vi "CMD_Loop.vi"() -> ()   [LabVIEW 2020, in "2023-Auto_CMD.lvlib"]
uses:
  2023-Auto_CMD.lvlib
  Cluster_CMD_CMD_Data.ctl
  Shared Code/TypeDefs/ENUM_AutoSelect.ctl
  Shared Code/TypeDefs/Cluster_Auto Sequence Data.ctl
  ENUM_CMD_State.ctl
  Shared Code/TypeDefs/Cluster_Auto Sequence Settings.ctl
  ENUM_Drive Mode Select.ctl
  Shared Code/TypeDefs/Dial_Compase heading unit circle CCW positive.ctl
  MotionMaser/ENUM_Pose List.ctl
  Shared Code/TypeDefs/ENUM_Grabber_CMD_Mode Select.ctl
  Shared Code/TypeDefs/Cluster_Extend_SW Output Data.ctl
  Shared Code/TypeDefs/Cluster_Sholder_SW Output Data.ctl
  Sholder/Cluster_CMD_ACT_Data.ctl
  Shared Code/TypeDefs/ENUM_Sholder_CMD_Mode Select.ctl
  SwerveDrive/Cluster_CMD_ACT_Data.ctl
  Shared Code/TypeDefs/ENUM_Swerve_CMD_Mode Select.ctl
  Shared Code/TypeDefs/Cluster_CMD_Direction Data.ctl
  Shared Code/TypeDefs/Cluster_Module Velocity-Direction-Rotations.ctl
  Shared Code/TypeDefs/Level_Velocity plus-minus 1.ctl
  Type Defs/NUM_Rotate Input.ctl
  Shared Code/TypeDefs/Cluster_X-Y.ctl
  Grabber/Cluster_CMD_ACT_Data.ctl
  Extention/Cluster_CMD_ACT_Data.ctl
  Shared Code/TypeDefs/ENUM_Extend_CMD_Mode Select.ctl
  Wrist/Cluster_CMD_ACT_Data.ctl
  Shared Code/TypeDefs/ENUM_Wrist_CMD_Mode Select.ctl
  PigeonIMU/Cluster_CMD_SEN_Data.ctl
  Shared Code/TypeDefs/Cluster_Wrist_SW Output Data.ctl
  ENUM_CMD_Action.ctl
  Shared Code/TypeDefs/Cluster_AutoSequence.ctl
  Type Defs/Cluster_Pigeon Tilt Data.ctl
  Shared Code/TypeDefs/ENUM_Tilt State.ctl
  Shared Code/TypeDefs/Cluster_Grabber_SW Outputs.ctl
  <vilib>/Rock Robotics/WPI/DriverStation/WPI_DriverStationRobotMode2.ctl
  Shared Code/TypeDefs/Cluster_Config_AutoData.ctl
  fdd46993-b9fc-440f-aafb-7ab1a8c35176.vi
  133b30be-2fcb-456e-b4b0-07f770c500ae.vi
  1ba0cf27-86ce-4142-8b65-bcb405614ff3.vi
  09229b25-3731-4416-b61c-801146eec302.vi
  c7d6c6c0-b27b-4b8b-8552-511dbe9cf3c3.vi
  dfaa9063-9cc7-40d1-a81d-c10c38088b54.vi
  fdd46993-b9fc-440f-aafb-7ab1a8c35176.vi/f38ca901-adc1-4ad8-996e-31aeb746ae36.vi
  fdd46993-b9fc-440f-aafb-7ab1a8c35176.vi/958b2683-dd4b-41b7-8ed1-41c95f63cef0.vi
  133b30be-2fcb-456e-b4b0-07f770c500ae.vi/f38ca901-adc1-4ad8-996e-31aeb746ae36.vi
  133b30be-2fcb-456e-b4b0-07f770c500ae.vi/958b2683-dd4b-41b7-8ed1-41c95f63cef0.vi
  09229b25-3731-4416-b61c-801146eec302.vi/f38ca901-adc1-4ad8-996e-31aeb746ae36.vi
  09229b25-3731-4416-b61c-801146eec302.vi/958b2683-dd4b-41b7-8ed1-41c95f63cef0.vi
  c7d6c6c0-b27b-4b8b-8552-511dbe9cf3c3.vi/f38ca901-adc1-4ad8-996e-31aeb746ae36.vi
  c7d6c6c0-b27b-4b8b-8552-511dbe9cf3c3.vi/958b2683-dd4b-41b7-8ed1-41c95f63cef0.vi
  fdd46993-b9fc-440f-aafb-7ab1a8c35176.vi/f38ca901-adc1-4ad8-996e-31aeb746ae36.vi/1c6bd52c-bbca-4d4a-a290-93ea2703fded.vi
  fdd46993-b9fc-440f-aafb-7ab1a8c35176.vi/f38ca901-adc1-4ad8-996e-31aeb746ae36.vi/47c2b0d5-b5fa-444e-9535-611565d375db.vi
  133b30be-2fcb-456e-b4b0-07f770c500ae.vi/f38ca901-adc1-4ad8-996e-31aeb746ae36.vi/1c6bd52c-bbca-4d4a-a290-93ea2703fded.vi
  133b30be-2fcb-456e-b4b0-07f770c500ae.vi/f38ca901-adc1-4ad8-996e-31aeb746ae36.vi/47c2b0d5-b5fa-444e-9535-611565d375db.vi
  09229b25-3731-4416-b61c-801146eec302.vi/f38ca901-adc1-4ad8-996e-31aeb746ae36.vi/1c6bd52c-bbca-4d4a-a290-93ea2703fded.vi
  09229b25-3731-4416-b61c-801146eec302.vi/f38ca901-adc1-4ad8-996e-31aeb746ae36.vi/47c2b0d5-b5fa-444e-9535-611565d375db.vi
  c7d6c6c0-b27b-4b8b-8552-511dbe9cf3c3.vi/f38ca901-adc1-4ad8-996e-31aeb746ae36.vi/1c6bd52c-bbca-4d4a-a290-93ea2703fded.vi
  c7d6c6c0-b27b-4b8b-8552-511dbe9cf3c3.vi/f38ca901-adc1-4ad8-996e-31aeb746ae36.vi/47c2b0d5-b5fa-444e-9535-611565d375db.vi
  Robot Global Data.vi
  Utility/Global_STOP.vi
  <vilib>/Utility/Data Type/Get Type Information.vi
  <vilib>/Utility/error.llb/Trim Whitespace.vi
  Shared Code/Utility/RWA/RWA/File/RWA_PC FIle Read String.vi
  Shared Code/Utility/RWA/RWA/Read Write Anything/RWA_File String.vi
  Shared Code/Utility/RWA/RWA/File/RWA_PC File Write String.vi
  Wrist/Global_CMD_ACT_Data In.vi
  Extention/Global_CMD_ACT_Data In.vi
  Grabber/Global_CMD_ACT_Data In.vi
  PigeonIMU/Global_CMD_SEN_Data In.vi
  SwerveDrive/Global_CMD_ACT_Data In.vi
  Sholder/Global_CMD_ACT_Data In.vi
  Global_CMD_CMD_Data In.vi
  Sholder/Global_ACT_Data Out.vi
  Extention/Global_ACT_Data Out.vi
  SwerveDrive/Global_ACT_Data Out.vi
  Grabber/Global_ACT_Data Out.vi
  Wrist/Global_ACT_Data Out.vi
  PigeonIMU/Global_SEN_Data Out.vi
  Global_CMD_Data Out.vi
  <vilib>/Comparison/Equal/Equal Functor/Equal Functor.lvclass
  PigeonIMU/PigeonIMU_SEN.lvlib
  Sholder/Sholder_ACT.lvlib
  SwerveDrive/SwerveDrive_ACT.lvlib
  Extention/Extend_ACT.lvlib
  Grabber/Grabber_ACT.lvlib
  Wrist/Wrist_ACT.lvlib
  MotionMaser/MotionMaster_SubCMD.lvlib
panel:
  out "Swerve_Position ft":dbl
  out "Remaing Match Time":sgl
  out "Sen_Pigeon_Tilt Data":T1
  out "Step Index 2":i32
  out "CMD Input.Auto Select":T3=enum."Drop Mid Drive Straight"
  out "Found":bool
  out "Error Out":errorcluster
  out "Message Out":string
  in  "Read Saved Config":bool
  in  "Update Config":bool
  in  "Sequences":T4[](array[typedef])=[{"Name"=enum."Score Mid Over and Balance", "List"=[{"State"=enum."Moving Arm", "Max Wait Time (S)"=1.5, "CMDs"={"Drive Mode"=enum."Coast", "Auto Angle"=0.0, "Auto Target (ft)"=0.0, "Max speed ft/s"=0.0, "Arm Pose "=enum."Safe Position", "Grabber CMD"=enum."STOP"}, "Color Box"=0}, {"State"=enum."Moving Arm", "Max Wait Time (S)"=3.0, "CMDs"={"Drive Mode"=enum."Coast", "Auto Angle"=0.0, "Auto Target (ft)"=0.0, "Max speed ft/s"=0.0, "Arm Pose "=enum."Score Mid", "Grabber CMD"=enum."STOP"}, "Color Box"=10309376}, {"State"=enum."Grabbing", "Max Wait Time (S)"=0.2, "CMDs"={"Drive Mode"=enum."To Position", "Auto Angle"=0.0, "Auto Target (ft)"=10.0, "Max speed ft/s"=12.0, "Arm Pose "=enum."Score Mid", "Grabber CMD"=enum."Eject"}, "Color Box"=16711680}, {"State"=enum."Tilt UP or Position", "Max Wait Time (S)"=8.0, "CMDs"={"Drive Mode"=enum."To Position", "Auto Angle"=0.5, "Auto Target (ft)"=6.0, "Max speed ft/s"=14.0, "Arm Pose "=enum."Home Pos", "Grabber CMD"=enum."STOP"}, "Color Box"=16744448}, {"State"=enum."Driving to Position", "Max Wait Time (S)"=10.0, "CMDs"={"Drive Mode"=enum."To Position", "Auto Angle"=0.5, "Auto Target (ft)"=14.0, "Max speed ft/s"=10.0, "Arm Pose "=enum."Home Pos", "Grabber CMD"=enum."STOP"}, "Color Box"=16776960}, {"State"=enum."Driving to Position", "Max Wait Time (S)"=3.0, "CMDs"={"Drive Mode"=enum."To Position", "Auto Angle"=0.0, "Auto Target (ft)"=6.0, "Max speed ft/s"=13.0, "Arm Pose "=enum."Home Pos", "Grabber CMD"=enum."STOP"}, "Color Box"=6618880}, {"State"=enum."Balancing Level", "Max Wait Time (S)"=100.0, "CMDs"={"Drive Mode"=enum."Balance on Charger", "Auto Angle"=0.0, "Auto Target (ft)"=0.0, "Max speed ft/s"=10.0, "Arm Pose "=enum."None-Unknown", "Grabber CMD"=enum."STOP"}, "Color Box"=16860}]}, {"Name"=enum."Drop Mid Drive Straight", "List"=[{"State"=enum."Moving Arm", "Max Wait Time (S)"=1.5, "CMDs"={"Drive Mode"=enum."Coast", "Auto Angle"=0.0, "Auto Target (ft)"=0.0, "Max speed ft/s"=0.0, "Arm Pose "=enum."Safe Position", "Grabber CMD"=enum."STOP"}, "Color Box"=0}, {"State"=enum."Moving Arm", "Max Wait Time (S)"=4.0, "CMDs"={"Drive Mode"=enum."Coast", "Auto Angle"=0.0, "Auto Target (ft)"=0.0, "Max speed ft/s"=0.0, "Arm Pose "=enum."Score Mid", "Grabber CMD"=enum."STOP"}, "Color Box"=10309376}, {"State"=enum."Grabbing", "Max Wait Time (S)"=0.5, "CMDs"={"Drive Mode"=enum."To Position", "Auto Angle"=0.0, "Auto Target (ft)"=0.0, "Max speed ft/s"=0.0, "Arm Pose "=enum."Score Mid", "Grabber CMD"=enum."Eject"}, "Color Box"=16711680}, {"State"=enum."Driving to Position", "Max Wait Time (S)"=10.0, "CMDs"={"Drive Mode"=enum."To Position", "Auto Angle"=0.5, "Auto Target (ft)"=15.0, "Max speed ft/s"=16.0, "Arm Pose "=enum."Safe Position", "Grabber CMD"=enum."STOP"}, "Color Box"=16744448}, {"State"=enum."Moving Arm", "Max Wait Time (S)"=10.0, "CMDs"={"Drive Mode"=enum."Rotation Absolute", "Auto Angle"=0.0, "Auto Target (ft)"=0.0, "Max speed ft/s"=0.0, "Arm Pose "=enum."Safe Position", "Grabber CMD"=enum."STOP"}, "Color Box"=16776960}]}, {"Name"=enum."Drop mid dock and engage", "List"=[{"State"=enum."Moving Arm", "Max Wait Time (S)"=1.5, "CMDs"={"Drive Mode"=enum."Coast", "Auto Angle"=0.0, "Auto Target (ft)"=0.0, "Max speed ft/s"=0.0, "Arm Pose "=enum."Safe Position", "Grabber CMD"=enum."STOP"}, "Color Box"=0}, {"State"=enum."Moving Arm", "Max Wait Time (S)"=4.0, "CMDs"={"Drive Mode"=enum."Coast", "Auto Angle"=0.0, "Auto Target (ft)"=0.0, "Max speed ft/s"=0.0, "Arm Pose "=enum."Score Mid", "Grabber CMD"=enum."STOP"}, "Color Box"=10309376}, {"State"=enum."Grabbing", "Max Wait Time (S)"=0.2, "CMDs"={"Drive Mode"=enum."Coast", "Auto Angle"=0.0, "Auto Target (ft)"=0.0, "Max speed ft/s"=0.0, "Arm Pose "=enum."Score Mid", "Grabber CMD"=enum."Eject"}, "Color Box"=16711680}, {"State"=enum."Driving to Position", "Max Wait Time (S)"=4.0, "CMDs"={"Drive Mode"=enum."To Position", "Auto Angle"=0.5, "Auto Target (ft)"=6.0, "Max speed ft/s"=10.0, "Arm Pose "=enum."Home Pos", "Grabber CMD"=enum."STOP"}, "Color Box"=16744448}, {"State"=enum."Balancing Level", "Max Wait Time (S)"=100.0, "CMDs"={"Drive Mode"=enum."Balance on Charger", "Auto Angle"=0.4996, "Auto Target (ft)"=0.0, "Max speed ft/s"=10.0, "Arm Pose "=enum."Home Pos", "Grabber CMD"=enum."STOP"}, "Color Box"=16776960}]}, {"Name"=enum."Drop High dock and engage", "List"=[{"State"=enum."Grabbing", "Max Wait Time (S)"=0.2, "CMDs"={"Drive Mode"=enum."Coast", "Auto Angle"=0.0, "Auto Target (ft)"=0.0, "Max speed ft/s"=0.0, "Arm Pose "=enum."Score Mid", "Grabber CMD"=enum."STOP"}, "Color Box"=0}, {"State"=enum."Driving to Position", "Max Wait Time (S)"=5.0, "CMDs"={"Drive Mode"=enum."To Position", "Auto Angle"=0.5, "Auto Target (ft)"=15.0, "Max speed ft/s"=10.0, "Arm Pose "=enum."Score High", "Grabber CMD"=enum."STOP"}, "Color Box"=10309376}, {"State"=enum."Driving to Position", "Max Wait Time (S)"=3.0, "CMDs"={"Drive Mode"=enum."Coast", "Auto Angle"=0.0, "Auto Target (ft)"=10.0, "Max speed ft/s"=16.0, "Arm Pose "=enum."Score High", "Grabber CMD"=enum."Eject"}, "Color Box"=16711680}, {"State"=enum."Balancing Level", "Max Wait Time (S)"=100.0, "CMDs"={"Drive Mode"=enum."To Position", "Auto Angle"=0.5, "Auto Target (ft)"=6.0, "Max speed ft/s"=16.0, "Arm Pose "=enum."Home Pos", "Grabber CMD"=enum."STOP"}, "Color Box"=16744448}, {"State"=enum."Idling", "Max Wait Time (S)"=5.0, "CMDs"={"Drive Mode"=enum."Coast", "Auto Angle"=0.0, "Auto Target (ft)"=0.0, "Max speed ft/s"=0.0, "Arm Pose "=enum."None-Unknown", "Grabber CMD"=enum."STOP"}, "Color Box"=16776960}]}, {"Name"=enum."Drop Low dock and engage", "List"=[{"State"=enum."Grabbing", "Max Wait Time (S)"=0.5, "CMDs"={"Drive Mode"=enum."Coast", "Auto Angle"=0.0, "Auto Target (ft)"=0.0, "Max speed ft/s"=0.0, "Arm Pose "=enum."Home Pos", "Grabber CMD"=enum."Eject"}, "Color Box"=0}, {"State"=enum."Driving to Position", "Max Wait Time (S)"=4.0, "CMDs"={"Drive Mode"=enum."To Position", "Auto Angle"=0.5, "Auto Target (ft)"=9.0, "Max speed ft/s"=10.0, "Arm Pose "=enum."Home Pos", "Grabber CMD"=enum."STOP"}, "Color Box"=10309376}, {"State"=enum."Balancing Level", "Max Wait Time (S)"=100.0, "CMDs"={"Drive Mode"=enum."Balance on Charger", "Auto Angle"=0.5, "Auto Target (ft)"=0.0, "Max speed ft/s"=5.0, "Arm Pose "=enum."Home Pos", "Grabber CMD"=enum."STOP"}, "Color Box"=16711680}]}, {"Name"=enum."Over and Rebalance", "List"=[{"State"=enum."Grabbing", "Max Wait Time (S)"=0.2, "CMDs"={"Drive Mode"=enum."Coast", "Auto Angle"=0.0, "Auto Target (ft)"=0.0, "Max speed ft/s"=0.0, "Arm Pose "=enum."Home Pos", "Grabber CMD"=enum."Eject"}, "Color Box"=0}, {"State"=enum."Tilt UP or Position", "Max Wait Time (S)"=8.0, "CMDs"={"Drive Mode"=enum."To Position", "Auto Angle"=0.5, "Auto Target (ft)"=6.0, "Max speed ft/s"=12.0, "Arm Pose "=enum."Home Pos", "Grabber CMD"=enum."STOP"}, "Color Box"=10309376}, {"State"=enum."Driving to Position", "Max Wait Time (S)"=10.0, "CMDs"={"Drive Mode"=enum."To Position", "Auto Angle"=0.5, "Auto Target (ft)"=14.0, "Max speed ft/s"=9.0, "Arm Pose "=enum."Home Pos", "Grabber CMD"=enum."STOP"}, "Color Box"=16711680}, {"State"=enum."Driving to Position", "Max Wait Time (S)"=3.0, "CMDs"={"Drive Mode"=enum."To Position", "Auto Angle"=0.0, "Auto Target (ft)"=6.0, "Max speed ft/s"=13.0, "Arm Pose "=enum."Home Pos", "Grabber CMD"=enum."STOP"}, "Color Box"=16744448}, {"State"=enum."Balancing Level", "Max Wait Time (S)"=100.0, "CMDs"={"Drive Mode"=enum."Balance on Charger", "Auto Angle"=0.0, "Auto Target (ft)"=0.0, "Max speed ft/s"=10.0, "Arm Pose "=enum."Home Pos", "Grabber CMD"=enum."STOP"}, "Color Box"=16776960}]}] {"List"."CMDs"."Auto Angle" scale format="%.3f"}
  out "Balanced":bool
  out "Action":T12
  out "State":T6
  out "ACT_Wrist_SW Out":T13
  out "CMD_SEN_Pigeon_CMD":T14
  out "CMD_ACT_Wrist":T15
  out "Drive At Angle":bool
  out "Step Index":i32
  out "CMD_CMD_2022-Auto_Data":T17={"Auto Select"=enum."Drop mid dock and engage"}
  out "CMD_ACT_Extend":T18
  out "CMD_ACT_Grabber":T20
  out "CMD_ACT_Drive":T21 {"Auto Angle" scale format="%.3f"; "Direction"."Rotate(Yaw) CCW 1 CW -1" scale=1.0..-1.0; "Direction"."Traverse"."Angle" scale format="%.3f"; "Direction"."Traverse"."Velocity" scale=-1.0..1.0 scale format="%.1f"}
  out "CMD_ACT_Shooter":T28={"Mode"=enum."STOP", "Position (counts)"=0, "Velocity (0-1)"=1.0}
  in  "Reset Sequence":bool
  out "Sholder_SW_Out":T30
  out "Drive At Position":bool
  out "Extend_SW_Out":T31
  in  "Reset All":bool
  in  "Set Manual":bool
  in  "Single Step":T5={"State"=enum."Starting", "Max Wait Time (S)"=0.0, "CMDs"={"Drive Mode"=enum."Coast", "Auto Angle"=0.0, "Auto Target (ft)"=0.0, "Max speed ft/s"=0.0, "Arm Pose "=enum."None-Unknown", "Grabber CMD"=enum."STOP"}, "Color Box"=16448250} caption="Current Step" {"CMDs"."Auto Angle" scale format="%.3f"}
  out "Input Data":T17={"Auto Select"=enum."Drop mid dock and engage"}
  out "Cycle Time (S)":dbl format="%.3g"
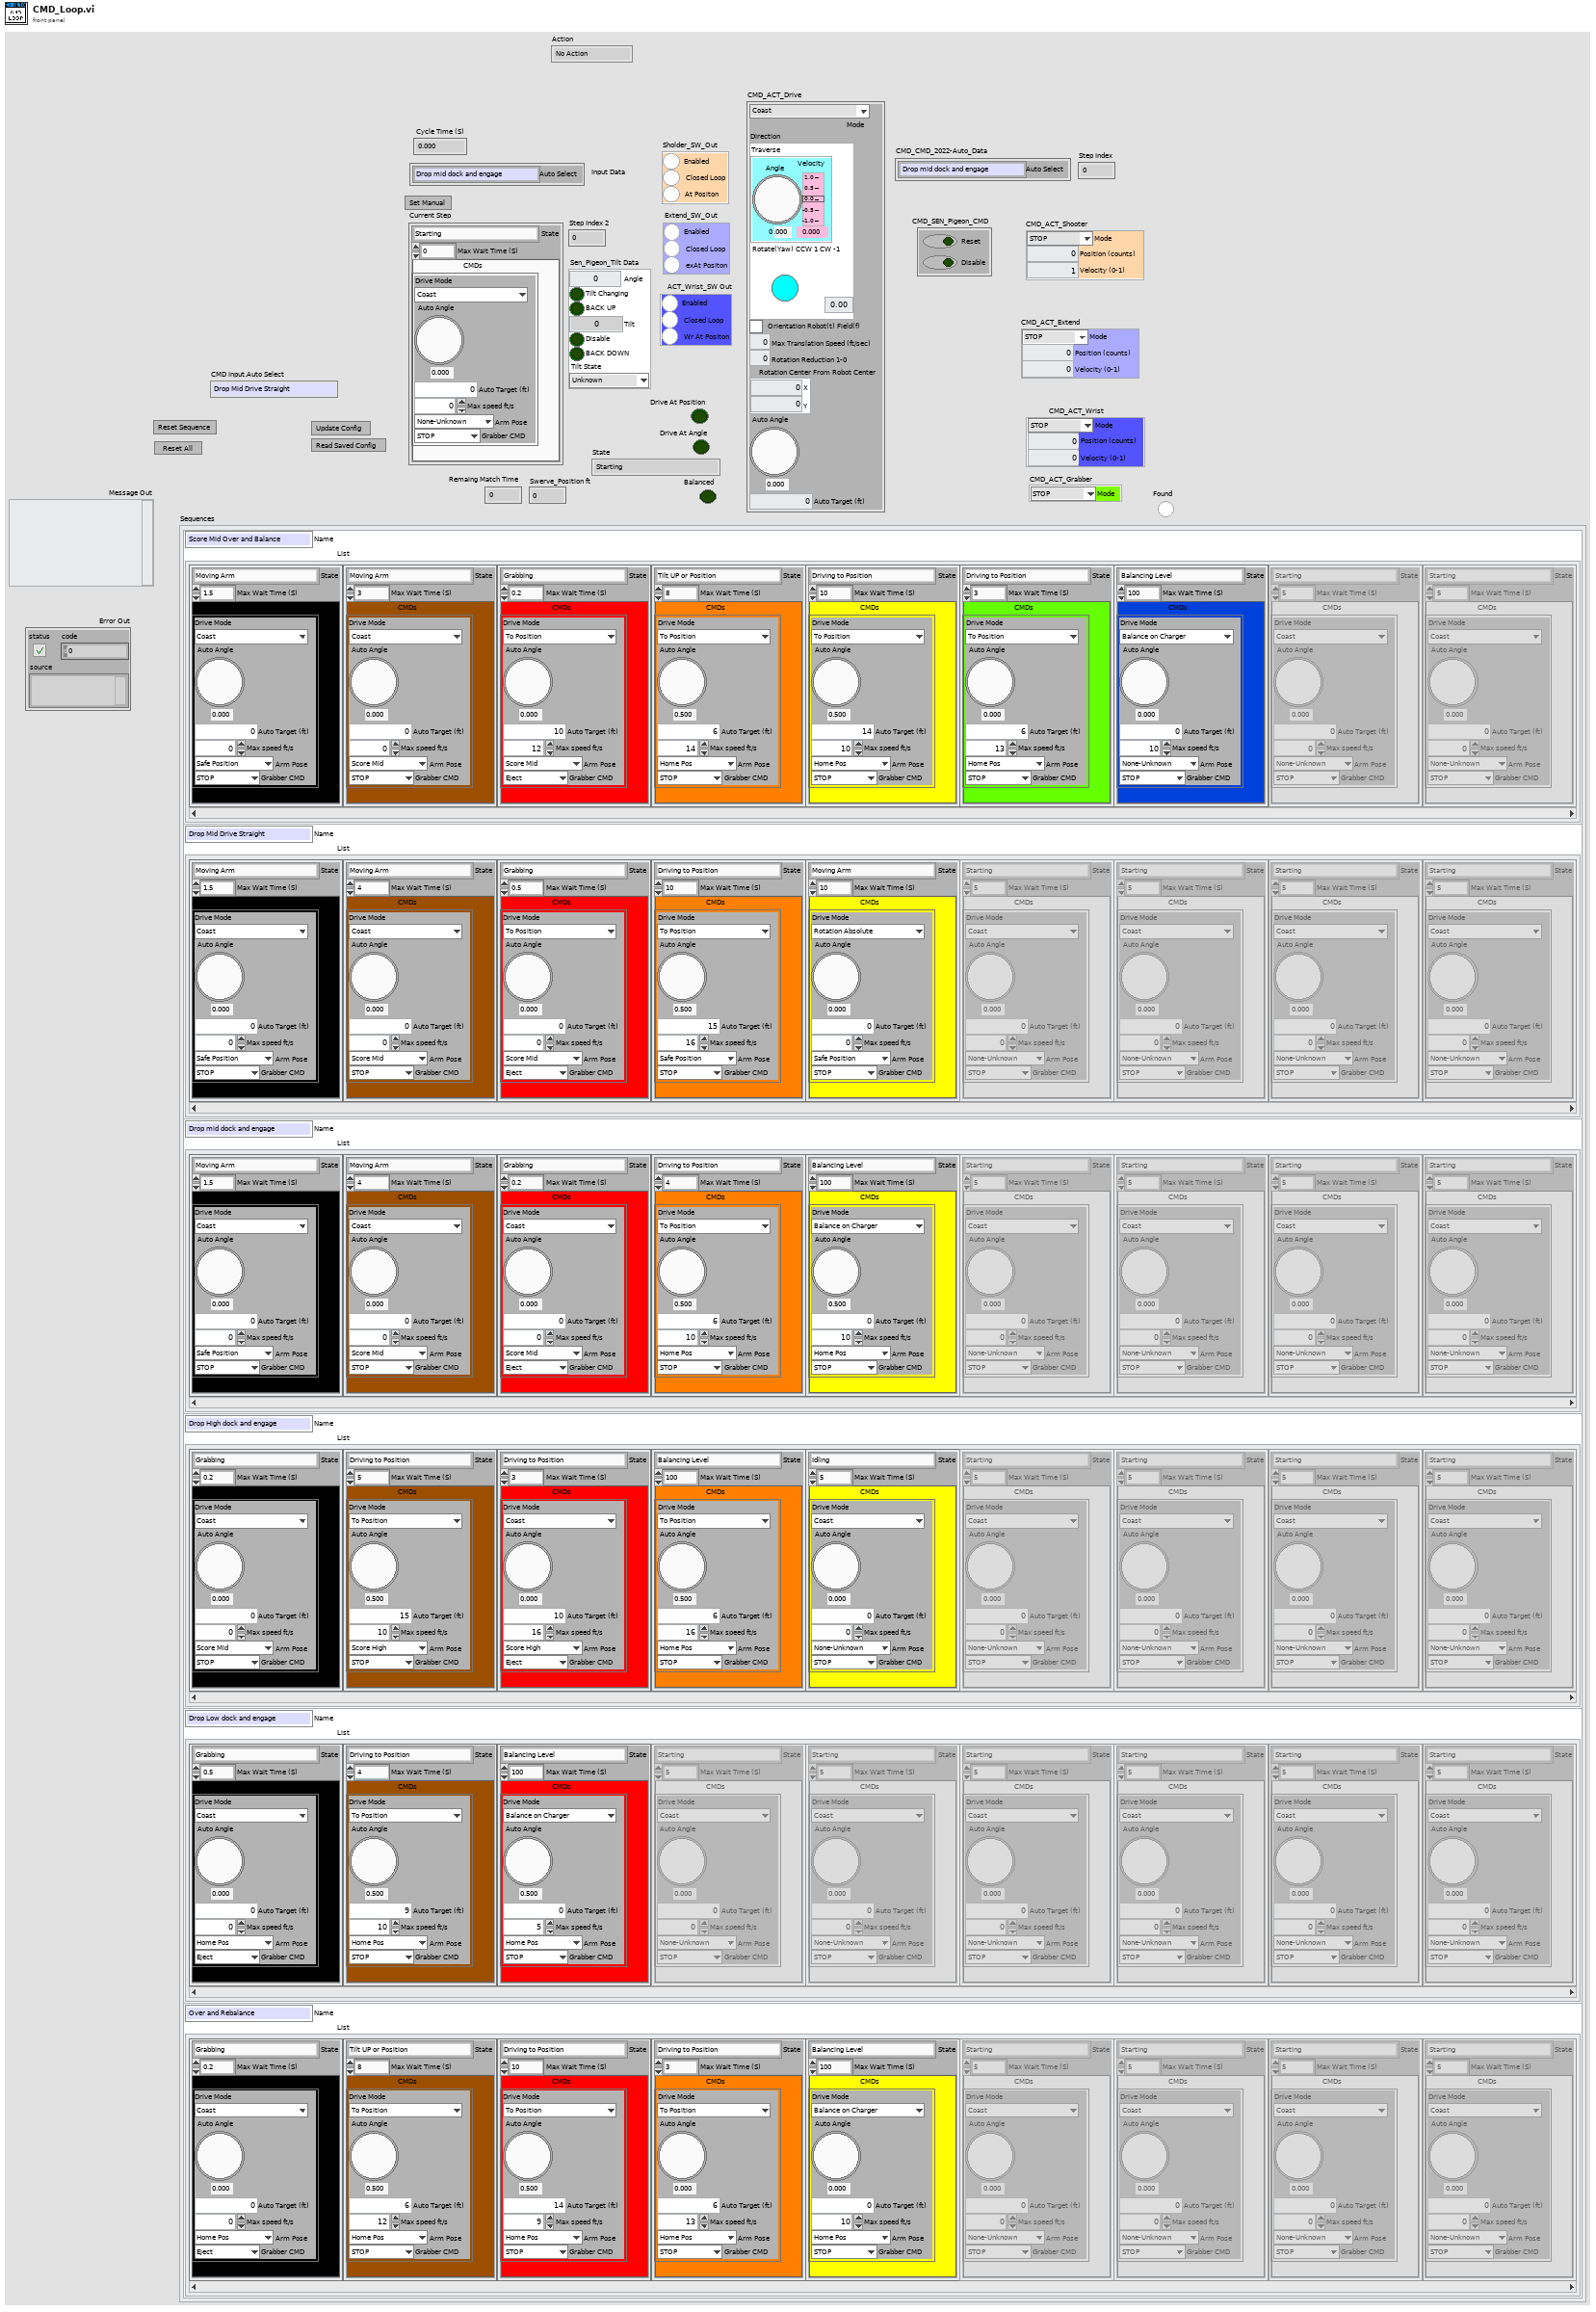
[diagram p1: front panel]
types:
  T1 = typedef "Cluster_Pigeon Tilt Data.ctl" = cluster{"Angle":dbl, "Tilt Changing":bool, "BACK UP":bool, "Tilt":dbl, "Disable":bool, "BACK DOWN":bool, "Tilt State":T2}
  T2 = typedef "ENUM_Tilt State.ctl" = enum16{"Unknown", "Level", "Angle UP from Level", "Level from Angle Up", "Angle Down from Level", "Level from Angle Down"}
  T3 = typedef "ENUM_AutoSelect.ctl" = enum16{"Unknown", "Drop Mid Drive Straight", "Drop mid dock and engage", "Drop High dock and engage", "Drop Low dock and engage", "Manual", "Over and Rebalance", "Over and Dock", "Score Mid Over and Balance", "Score High Over and Balance", "Score Mid ONLY", "Score High ONLY"}
  T4 = typedef "Cluster_AutoSequence.ctl" = cluster{"Name":T3, "List":T5[]}
  T5 = typedef "Cluster_Auto Sequence Data.ctl" = cluster{"State":T6, "Max Wait Time (S)":dbl, "CMDs":T7, "Color Box":u32}
  T6 = typedef "2023-Auto_CMD.lvlib/ENUM_CMD_State.ctl" = enum16{"Starting", "Idling", "Selecting Sequence", "Selecting Next Step", "Driving to Position", "Stopping", "Grabbing", "Moving Arm", "Rotation Target", "Waiting", "Shutting Down", "Balancing Level", "Configuring", "Tilt UP or Position", "Tile DOWN or Position", "LEVEL or Position"}
  T7 = typedef "Cluster_Auto Sequence Settings.ctl" = cluster{"Drive Mode":T8, "Auto Angle":T9, "Auto Target (ft)":dbl, "Max speed ft/s":dbl, "Arm Pose ":T10, "Grabber CMD":T11}
  T8 = typedef "2023-Auto_CMD.lvlib/ENUM_Drive Mode Select.ctl" = enum16{"Coast", "To Position", "Rotation Absolute", "Balance on Charger", "Brake", "Lock"}
  T9 = typedef "Dial_Compase heading unit circle CCW positive.ctl" = dbl
  T10 = typedef "MotionMaster_SubCMD.lvlib/ENUM_Pose List.ctl" = enum16{"None-Unknown", "Intake", "Score High", "Score Mid", "Safe Position", "Home Pos"}
  T11 = typedef "ENUM_Grabber_CMD_Mode Select.ctl" = enum16{"STOP", "Intake", "Eject"}
  T12 = typedef "2023-Auto_CMD.lvlib/ENUM_CMD_Action.ctl" = enum16{"No Action", "Reset Time", "Reset All", "Set System Cmds", "Reset Sequence", "Conveyor Off", "Config File Read", "Config File Wirte", "Config from FP", "Lock Wheels"}
  T13 = typedef "Cluster_Wrist_SW Output Data.ctl" = cluster{"Enabled":bool, "Closed Loop":bool, "Wr At Positon":bool}
  T14 = typedef "PigeonIMU_SEN.lvlib/Cluster_CMD_SEN_Data.ctl" = cluster{"Reset":bool, "Disable":bool}
  T15 = typedef "Wrist_ACT.lvlib/Cluster_CMD_ACT_Data.ctl" = cluster{"Mode":T16, "Position (counts)":i32, "Velocity (0-1)":dbl}
  T16 = typedef "ENUM_Wrist_CMD_Mode Select.ctl" = enum16{"STOP", "Position", "Speed"}
  T17 = typedef "2023-Auto_CMD.lvlib/Cluster_CMD_CMD_Data.ctl" = cluster{"Auto Select":T3}
  T18 = typedef "Extend_ACT.lvlib/Cluster_CMD_ACT_Data.ctl" = cluster{"Mode":T19, "Position (counts)":i32, "Velocity (0-1)":dbl}
  T19 = typedef "ENUM_Extend_CMD_Mode Select.ctl" = enum16{"STOP", "Position", "Velocity", "Force Home"}
  T20 = typedef "Grabber_ACT.lvlib/Cluster_CMD_ACT_Data.ctl" = cluster{"Mode":T11}
  T21 = typedef "SwerveDrive_ACT.lvlib/Cluster_CMD_ACT_Data.ctl" = cluster{"Mode":T22, "Direction":T23, "Orientation Robot(t) Field(f)":bool, "Max Translation Speed (ft/sec)":dbl, "Rotation Reduction 1-0":dbl, "Rotation Center From Robot Center":T27, "Auto Angle":T9, "Auto Target (ft)":dbl}
  T22 = typedef "ENUM_Swerve_CMD_Mode Select.ctl" = enum16{"Coast", "Manual", "Auto Trans Auto Rotate", "Manual Trans Auto Rotate", "Balance", "Stop Brake", "Lock Wheels"}
  T23 = typedef "Cluster_CMD_Direction Data.ctl" = cluster{"Traverse":T24, "Rotate(Yaw) CCW 1 CW -1":T26}
  T24 = typedef "Cluster_Module Velocity-Direction-Rotations.ctl" = cluster{"Velocity":T25, "Angle":T9, "Rotations Count":dbl}
  T25 = typedef "Level_Velocity plus-minus 1.ctl" = dbl
  T26 = typedef "NUM_Rotate Input.ctl" = dbl
  T27 = typedef "Cluster_X-Y.ctl" = cluster{"X":dbl, "Y":dbl}
  T28 = typedef "Sholder_ACT.lvlib/Cluster_CMD_ACT_Data.ctl" = cluster{"Mode":T29, "Position (counts)":i32, "Velocity (0-1)":dbl}
  T29 = typedef "ENUM_Sholder_CMD_Mode Select.ctl" = enum16{"STOP", "Position", "Percent out"}
  T30 = typedef "Cluster_Sholder_SW Output Data.ctl" = cluster{"Enabled":bool, "Closed Loop":bool, "At Positon":bool}
  T31 = typedef "Cluster_Extend_SW Output Data.ctl" = cluster{"Enabled":bool, "Closed Loop":bool, "exAt Positon":bool}
  T32 = typedef "Cluster_Config_AutoData.ctl" = cluster{"AutoData Ver":u64, "Sequences":T4[]}
  T33 = typedef "WPI_DriverStationRobotMode2.ctl" = enum16{"Autonomous Disabled", "Autonomous Enabled", "Teleop Disabled", "Teleop Enabled", "Disconnected", "Finish", "Test Disabled", "Test Enabled", "Emergency Stopped"}
  T34 = typedef "Cluster_Grabber_SW Outputs.ctl" = cluster{"Enabled":bool, "Closed Loop":bool, "Stalled":bool}
  T35 = cluster{"State":T6, "Previous State":T6, "Current Time":timestamp, "Previous Time":timestamp, "Start Time":timestamp, "Target Time (ms)":u32, "Cycle Time(S)":dbl, "CMD Input":T17, "CMD_ACT_Sholder":T28, "CMD_ACT_SwerveDrive":T21, "CMD_SEN_Pigeon_CMD":T14, "Sholder_SW_Outputs":T30, "SwerveDrive_Directions":dbl[], "CMD_ACT_Grabber":T20, "Grabber_SW_Out":T34, "Wrist_SW_Out":T13, "CMD_ACT_Extend":T18, "Sequence Array":T5[], "Step Data":T7, "Step Index":i32, "Drive At Position":bool, "Extend_SW_Out":T31, "Robot Mode":T33, "Prev Robot Mode":T33, "Auto Select ":T3, "At Angle Target":bool, "CMD_ACT_Wrist_Data":T15, "Balanced":bool, "Team Files Folder":path, "AutoData":T32, "Update Display":bool, "Data Read":bool, "Tilt Data":T1, "Remaing Match Time":sgl, "Swerve_Position ft":dbl}
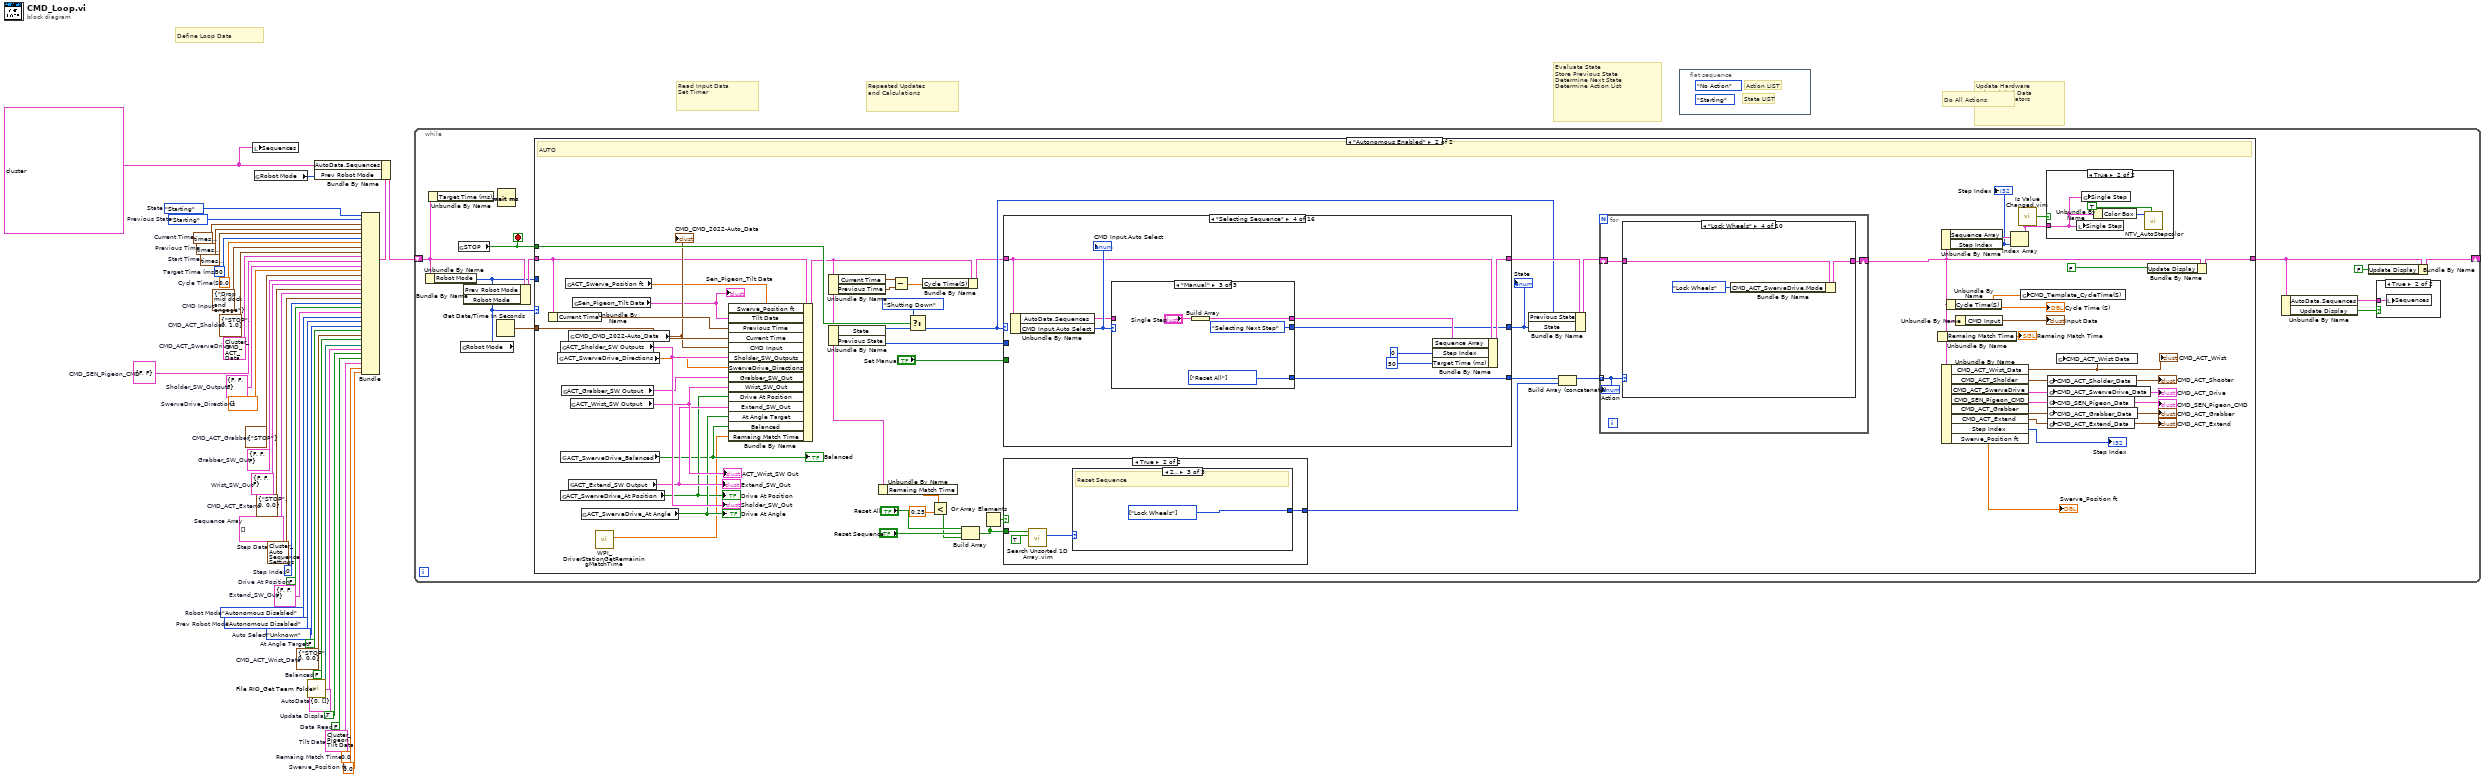
[diagram p0: block diagram]
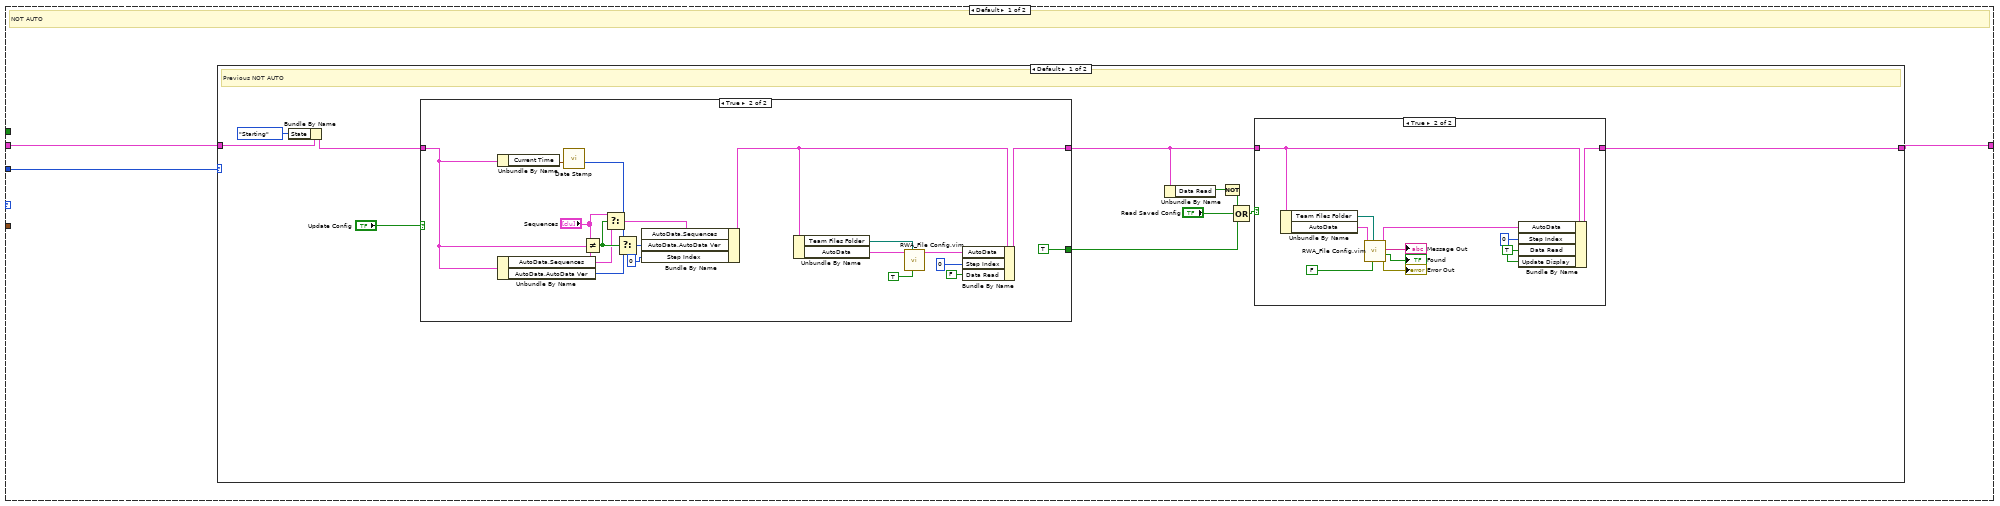
[diagram p3: hidden frame]
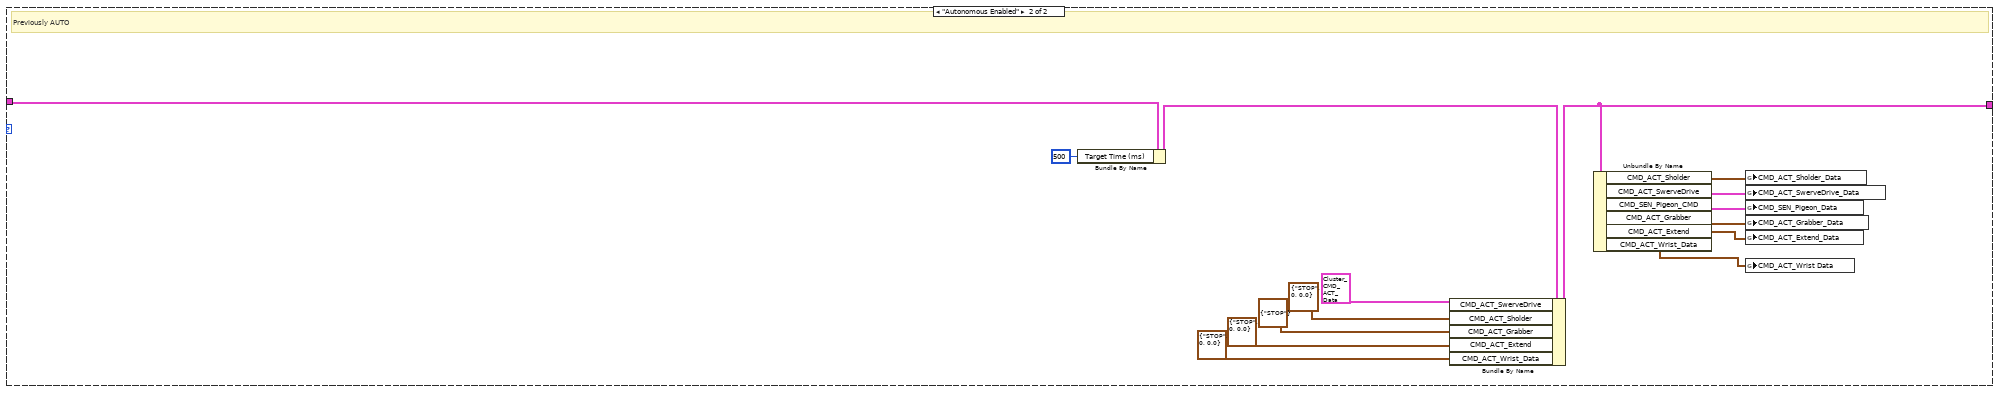
[diagram p6: hidden frame]
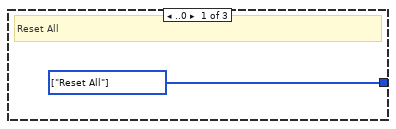
[diagram p8: hidden frame]
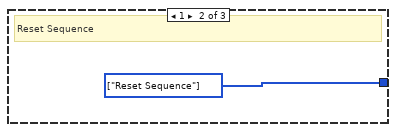
[diagram p9: hidden frame]
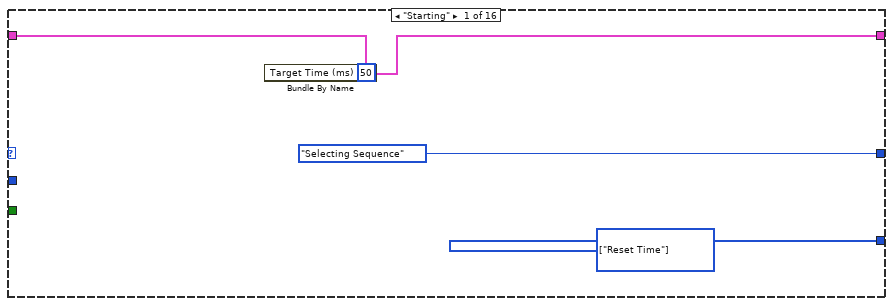
[diagram p10: hidden frame]
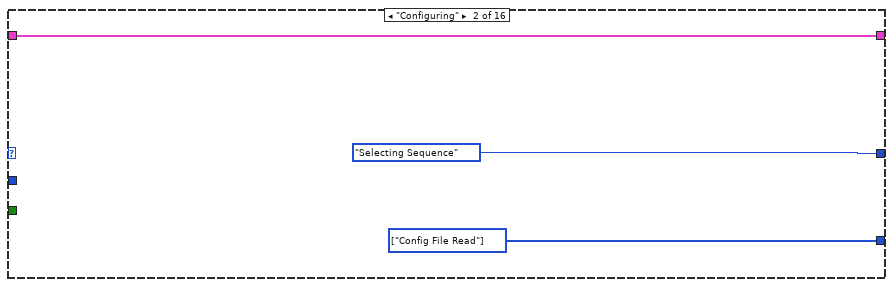
[diagram p11: hidden frame]
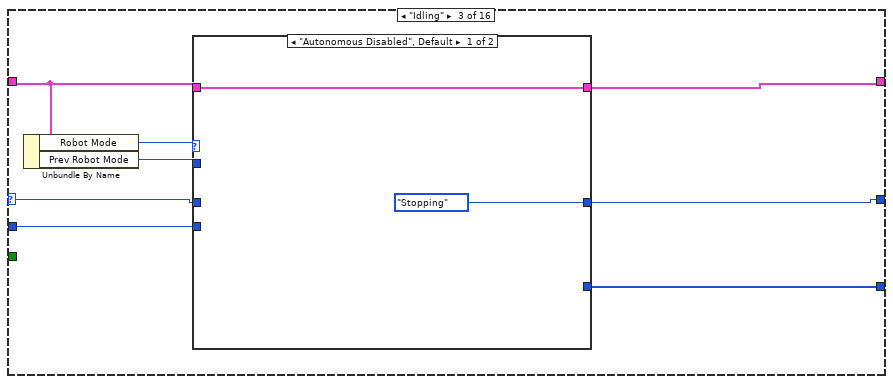
[diagram p12: hidden frame]
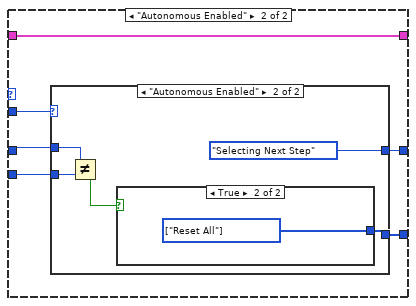
[diagram p13: hidden frame]
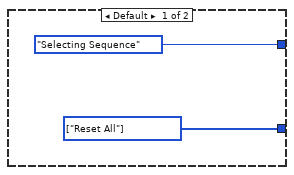
[diagram p14: hidden frame]
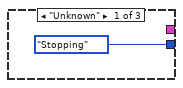
[diagram p16: hidden frame]
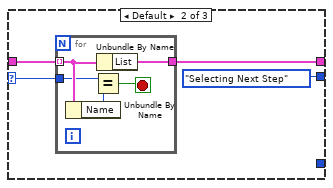
[diagram p17: hidden frame]
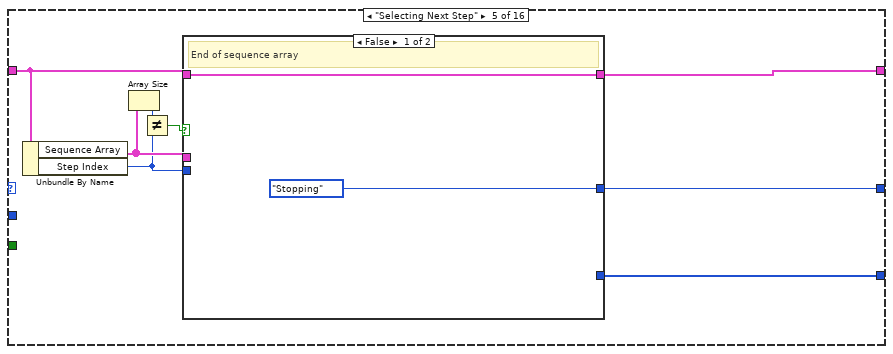
[diagram p18: hidden frame]
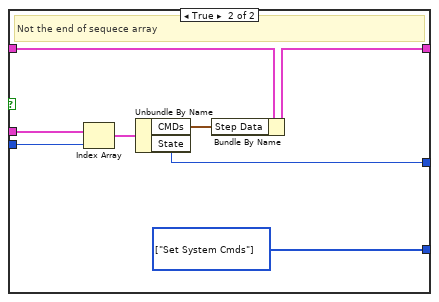
[diagram p19: hidden frame]
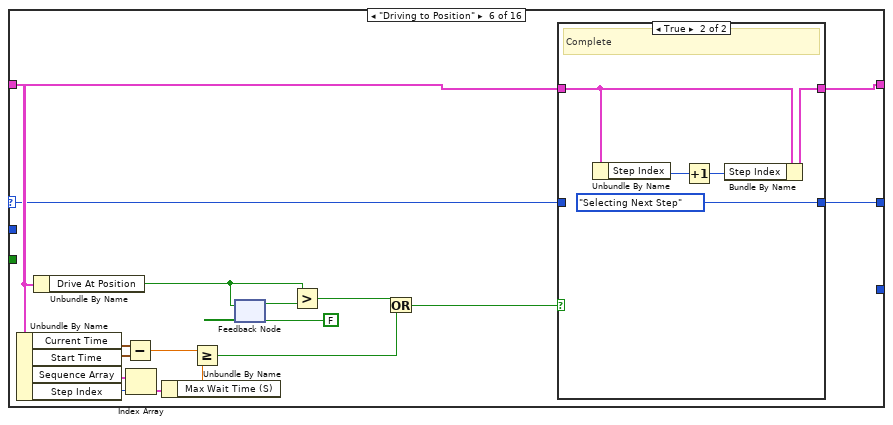
[diagram p20: hidden frame]
diagram:
  w1 = 0.0  # Swerve_Position ft
  w2 = sgl 0.0  # Remaing Match Time
  w3 = T1 {"Angle"=0.00439453125, "Tilt Changing"=FALSE, "BACK UP"=FALSE, "Tilt"=0.0, "Disable"=FALSE, "BACK DOWN"=FALSE, "Tilt State"=enum."Unknown"}  # Tilt Data
  w4 = T4[] [{"Name"=enum."Drop Mid Drive Straight", "List"=[{"State"=enum."Moving Arm", "Max Wait Time (S)"=1.5, "CMDs"={"Drive Mode"=enum."Coast", "Auto Angle"=0.0, "Auto Target (ft)"=0.0, "Max speed ft/s"=0.0, "Arm Pose "=enum."Safe Position", "Grabber CMD"=enum."STOP"}, "Color Box"=16448250}, {"State"=enum."Moving Arm", "Max Wait Time (S)"=4.0, "CMDs"={"Drive Mode"=enum."Coast", "Auto Angle"=0.0, "Auto Target (ft)"=0.0, "Max speed ft/s"=0.0, "Arm Pose "=enum."Score Mid", "Grabber CMD"=enum."STOP"}, "Color Box"=16448250}, {"State"=enum."Grabbing", "Max Wait Time (S)"=0.5, "CMDs"={"Drive Mode"=enum."To Position", "Auto Angle"=0.0, "Auto Target (ft)"=0.0, "Max speed ft/s"=0.0, "Arm Pose "=enum."Score Mid", "Grabber CMD"=enum."Eject"}, "Color Box"=16448250}, {"State"=enum."Driving to Position", "Max Wait Time (S)"=10.0, "CMDs"={"Drive Mode"=enum."To Position", "Auto Angle"=0.5, "Auto Target (ft)"=15.0, "Max speed ft/s"=16.0, "Arm Pose "=enum."Safe Position", "Grabber CMD"=enum."STOP"}, "Color Box"=16448250}, {"State"=enum."Moving Arm", "Max Wait Time (S)"=10.0, "CMDs"={"Drive Mode"=enum."Coast", "Auto Angle"=0.0, "Auto Target (ft)"=0.0, "Max speed ft/s"=0.0, "Arm Pose "=enum."Safe Position", "Grabber CMD"=enum."STOP"}, "Color Box"=16448250}]}, {"Name"=enum."Drop mid dock and engage", "List"=[{"State"=enum."Moving Arm", "Max Wait Time (S)"=1.5, "CMDs"={"Drive Mode"=enum."Coast", "Auto Angle"=0.0, "Auto Target (ft)"=0.0, "Max speed ft/s"=0.0, "Arm Pose "=enum."Safe Position", "Grabber CMD"=enum."STOP"}, "Color Box"=16448250}, {"State"=enum."Moving Arm", "Max Wait Time (S)"=4.0, "CMDs"={"Drive Mode"=enum."Coast", "Auto Angle"=0.0, "Auto Target (ft)"=0.0, "Max speed ft/s"=0.0, "Arm Pose "=enum."Score Mid", "Grabber CMD"=enum."STOP"}, "Color Box"=16448250}, {"State"=enum."Grabbing", "Max Wait Time (S)"=0.2, "CMDs"={"Drive Mode"=enum."Coast", "Auto Angle"=0.0, "Auto Target (ft)"=0.0, "Max speed ft/s"=0.0, "Arm Pose "=enum."Score Mid", "Grabber CMD"=enum."Eject"}, "Color Box"=16448250}, {"State"=enum."Driving to Position", "Max Wait Time (S)"=4.0, "CMDs"={"Drive Mode"=enum."To Position", "Auto Angle"=0.5, "Auto Target (ft)"=6.0, "Max speed ft/s"=10.0, "Arm Pose "=enum."Home Pos", "Grabber CMD"=enum."STOP"}, "Color Box"=16448250}, {"State"=enum."Balancing Level", "Max Wait Time (S)"=100.0, "CMDs"={"Drive Mode"=enum."Balance on Charger", "Auto Angle"=0.4996, "Auto Target (ft)"=0.0, "Max speed ft/s"=10.0, "Arm Pose "=enum."Home Pos", "Grabber CMD"=enum."STOP"}, "Color Box"=16448250}]}, {"Name"=enum."Drop High dock and engage", "List"=[{"State"=enum."Moving Arm", "Max Wait Time (S)"=2.0, "CMDs"={"Drive Mode"=enum."Coast", "Auto Angle"=0.0, "Auto Target (ft)"=0.0, "Max speed ft/s"=0.0, "Arm Pose "=enum."Score Mid", "Grabber CMD"=enum."STOP"}, "Color Box"=16448250}, {"State"=enum."Moving Arm", "Max Wait Time (S)"=3.0, "CMDs"={"Drive Mode"=enum."Coast", "Auto Angle"=0.0, "Auto Target (ft)"=0.0, "Max speed ft/s"=0.0, "Arm Pose "=enum."Score High", "Grabber CMD"=enum."STOP"}, "Color Box"=16448250}, {"State"=enum."Grabbing", "Max Wait Time (S)"=0.2, "CMDs"={"Drive Mode"=enum."Coast", "Auto Angle"=0.0, "Auto Target (ft)"=0.0, "Max speed ft/s"=0.0, "Arm Pose "=enum."Score High", "Grabber CMD"=enum."Eject"}, "Color Box"=16448250}, {"State"=enum."Driving to Position", "Max Wait Time (S)"=2.0, "CMDs"={"Drive Mode"=enum."To Position", "Auto Angle"=0.5, "Auto Target (ft)"=6.0, "Max speed ft/s"=16.0, "Arm Pose "=enum."Home Pos", "Grabber CMD"=enum."STOP"}, "Color Box"=16448250}, {"State"=enum."Balancing Level", "Max Wait Time (S)"=100.0, "CMDs"={"Drive Mode"=enum."Balance on Charger", "Auto Angle"=0.4996, "Auto Target (ft)"=0.0, "Max speed ft/s"=10.0, "Arm Pose "=enum."Home Pos", "Grabber CMD"=enum."STOP"}, "Color Box"=16448250}]}, {"Name"=enum."Drop Low dock and engage", "List"=[{"State"=enum."Grabbing", "Max Wait Time (S)"=0.5, "CMDs"={"Drive Mode"=enum."Coast", "Auto Angle"=0.0, "Auto Target (ft)"=0.0, "Max speed ft/s"=0.0, "Arm Pose "=enum."Home Pos", "Grabber CMD"=enum."Eject"}, "Color Box"=16448250}, {"State"=enum."Driving to Position", "Max Wait Time (S)"=4.0, "CMDs"={"Drive Mode"=enum."To Position", "Auto Angle"=0.5, "Auto Target (ft)"=9.0, "Max speed ft/s"=10.0, "Arm Pose "=enum."Home Pos", "Grabber CMD"=enum."STOP"}, "Color Box"=16448250}, {"State"=enum."Balancing Level", "Max Wait Time (S)"=100.0, "CMDs"={"Drive Mode"=enum."Balance on Charger", "Auto Angle"=0.5, "Auto Target (ft)"=0.0, "Max speed ft/s"=5.0, "Arm Pose "=enum."Home Pos", "Grabber CMD"=enum."STOP"}, "Color Box"=16448250}]}, {"Name"=enum."Over and Rebalance", "List"=[{"State"=enum."Grabbing", "Max Wait Time (S)"=0.5, "CMDs"={"Drive Mode"=enum."Coast", "Auto Angle"=0.0, "Auto Target (ft)"=0.0, "Max speed ft/s"=0.0, "Arm Pose "=enum."Home Pos", "Grabber CMD"=enum."Eject"}, "Color Box"=16448250}, {"State"=enum."Driving to Position", "Max Wait Time (S)"=8.0, "CMDs"={"Drive Mode"=enum."To Position", "Auto Angle"=0.5, "Auto Target (ft)"=15.0, "Max speed ft/s"=12.0, "Arm Pose "=enum."Home Pos", "Grabber CMD"=enum."STOP"}, "Color Box"=16448250}]}] ("Sequences")
  w5 = FALSE  # Data Read
  w6 = TRUE  # Update Display
  w7 = T32 {"AutoData Ver"=0, "Sequences"=[]}  # AutoData
  w9 = FALSE  # Balanced
  w10 = T15 {"Mode"=enum."STOP", "Position (counts)"=0, "Velocity (0-1)"=0.0}  # CMD_ACT_Wrist_Data
  w11 = FALSE  # At Angle Target
  w12 = ENUM_AutoSelect."Unknown"  # Auto Select
  w16 = WPI_DriverStationRobotMode2."Autonomous Disabled"  # Prev Robot Mode
  w17 = WPI_DriverStationRobotMode2."Autonomous Disabled"  # Robot Mode
  w18 = T31 {"Enabled"=FALSE, "Closed Loop"=FALSE, "exAt Positon"=FALSE}  # Extend_SW_Out
  w19 = FALSE  # Drive At Position
  w20 = 0  # Step Index
  w21 = T7 {"Drive Mode"=enum."Coast", "Auto Angle"=0.0, "Auto Target (ft)"=0.0, "Max speed ft/s"=0.0, "Arm Pose "=enum."None-Unknown", "Grabber CMD"=enum."STOP"}  # Step Data
  w22 = T5[] []  # Sequence Array
  w23 = T18 {"Mode"=enum."STOP", "Position (counts)"=0, "Velocity (0-1)"=0.0}  # CMD_ACT_Extend
  w24 = T13 {"Enabled"=FALSE, "Closed Loop"=FALSE, "Wr At Positon"=FALSE}  # Wrist_SW_Out
  w25 = dbl[] []  # SwerveDrive_Directions
  w26 = T30 {"Enabled"=FALSE, "Closed Loop"=FALSE, "At Positon"=FALSE}  # Sholder_SW_Outputs
  w27 = T34 {"Enabled"=FALSE, "Closed Loop"=FALSE, "Stalled"=FALSE}  # Grabber_SW_Out
  w28 = T20 {"Mode"=enum."STOP"}  # CMD_ACT_Grabber
  w29 = T14 {"Reset"=FALSE, "Disable"=FALSE}  # CMD_SEN_Pigeon_CMD
  w30 = T21 {"Mode"=enum."Coast", "Direction"={"Traverse"={"Velocity"=0.0, "Angle"=0.0, "Rotations Count"=0.0}, "Rotate(Yaw) CCW 1 CW -1"=0.0}, "Orientation Robot(t) Field(f)"=FALSE, "Max Translation Speed (ft/sec)"=0.0, "Rotation Reduction 1-0"=0.0, "Rotation Center From Robot Center"={"X"=0.0, "Y"=0.0}, "Auto Angle"=0.0, "Auto Target (ft)"=0.0}  # CMD_ACT_SwerveDrive
  w31 = T28 {"Mode"=enum."STOP", "Position (counts)"=0, "Velocity (0-1)"=1.0}  # CMD_ACT_Sholder
  w32 = 0.0  # Cycle Time(S)
  w33 = ENUM_CMD_State."Starting"  # Previous State
  w34 = timestamp(0 s since 1904-01-01)  # Previous Time
  w35 = u32 50  # Target Time (ms)
  w36 = T17 {"Auto Select"=enum."Drop mid dock and engage"}  # CMD Input
  w37 = timestamp(0 s since 1904-01-01)  # Start Time
  w38 = timestamp(0 s since 1904-01-01)  # Current Time
  w39 = ENUM_CMD_State."Starting"  # State
  # "Define Loop Data"
  # "Repeated Updates\nand Calculations"
  # "Read Input Data\nSet Timer"
  # "Evaluate State\nStore Previous State\nDetermine Next State\nDetermine Action List"
  # "Do All Actions"
  # "Update Hardware\nWrite Global Data\nUpdate Indicators"
  n1 = local write "Sequences"(w4) -> ()
  n2 = global read "Robot Global Data.vi" "Robot Mode"() -> (w13:T33)
  n3 = call "File RIO_Get Team Folder.vi"() -> ("Team Files Folder"=w8:path)  [unwired: 10 in, 1 out]
  n4 = Bundle("State"=w39, "Previous State"=w33, "Current Time"=w38, "Previous Time"=w34, "Start Time"=w37, "Target Time (ms)"=w35, "Cycle Time(S)"=w32, "CMD Input"=w36, "CMD_ACT_Sholder"=w31, "CMD_ACT_SwerveDrive"=w30, "CMD_SEN_Pigeon_CMD"=w29, "Sholder_SW_Outputs"=w26, "SwerveDrive_Directions"=w25, "CMD_ACT_Grabber"=w28, "Grabber_SW_Out"=w27, "Wrist_SW_Out"=w24, "CMD_ACT_Extend"=w23, "Sequence Array"=w22, "Step Data"=w21, "Step Index"=w20, "Drive At Position"=w19, "Extend_SW_Out"=w18, "Robot Mode"=w17, "Prev Robot Mode"=w16, "Auto Select"=w12, "At Angle Target"=w11, "CMD_ACT_Wrist_Data"=w10, "Balanced"=w9, "Team Files Folder"=w8, "AutoData"=w7, "Update Display"=w6, "Data Read"=w5, "Tilt Data"=w3, "Remaing Match Time"=w2, "Swerve_Position ft"=w1) -> (w15:T35)  [unwired: 1 in]
  n5 = Bundle By Name(cluster=w15, "AutoData.Sequences"=w4, "Prev Robot Mode"=w13) -> (w14:T35)
  n6 = while {
    shift-right: [w41] -> _
    shift-left: w14 -> [w48]
    stop <- w49 stop-if-true
    n7 = Unbundle By Name(w48) -> ("Robot Mode"=w46:T33)
    n8 = Unbundle By Name(w48) -> ("Target Time (ms)"=w50:u32)
    n9 = global read "Global_STOP.vi" "STOP"() -> (w49:bool)
    n10 = global read "Robot Global Data.vi" "Robot Mode"() -> (w45:T33)
    n11 = Bundle By Name(cluster=w48, "Prev Robot Mode"=w46, "Robot Mode"=w45) -> (w47:T35)
    n12 = Get Date/Time In Seconds() -> (seconds since 1Jan1904=w51:timestamp)
    n13 = Wait (ms)(milliseconds to wait=w50) -> ()  [unwired: 1 out]
    n14 = case shown="\"Autonomous Enabled\"" w45 {
      tunnel: w51 -> [_ w170]
      tunnel: [w54 w131] -> w42
      tunnel: w47 -> [w55 w124]
      tunnel: w46 -> [w53 _]
      tunnel: w49 -> [_ w143]
      frame Default {
        # "NOT AUTO"
        n15 = case shown="Default" w53 {
          tunnel: w55 -> [w66 w99]
          tunnel: [w60 w106] -> w54
          frame Default {
            # "Previous NOT AUTO"
            n16 = Bundle By Name(cluster=w66, "State"=ENUM_CMD_State."Starting") -> (w58:T35)
            n17 = case shown="True" "Update Config" {
              tunnel: w58 -> [w67 w77]
              tunnel: [w67 w69] -> w57
              tunnel: [_ TRUE] -> w56
              frame False {
              }
              frame True {
                n18 = Unbundle By Name(w77) -> ("AutoData.Sequences"=w80:T4[], "AutoData.AutoData Ver"=w84:u64)
                n19 = Unbundle By Name(w77) -> ("Current Time"=w86:timestamp)
                n20 = call "Date Stamp.vi"("Time"=w86) -> ("U64 Out"=w85:u64)  [unwired: 5 in, 1 out]
                n21 = Not Equal?(x="Sequences", y=w80) -> (x != y?=w82:bool)
                n22 = Select(t="Sequences", s=w82, f=w80) -> (s? t:f=w79:T4[])
                n23 = Select(t=w85, s=w82, f=w84) -> (s? t:f=w83:u64)
                n24 = Bundle By Name(cluster=w77, "AutoData.Sequences"=w79, "AutoData.AutoData Ver"=w83, "Step Index"=0) -> (w70:T35)
                n25 = Unbundle By Name(w70) -> ("Team Files Folder"=w75:path, "AutoData"=w74:T32)
                n26 = call "RWA_File Config.vim"("Read(f) Write(t)"=TRUE, "Target Folder Folder"=w75, "Any Config"=w74) -> ("Any Config Out"=w76:T32)  [unwired: 4 in, 4 out]
                n27 = Bundle By Name(cluster=w70, "AutoData"=w76, "Step Index"=0, "Data Read"=FALSE) -> (w69:T35)
              }
            }
            n28 = Unbundle By Name(w57) -> ("Data Read"=w64:bool)
            n29 = Not(x=w64) -> (.not. x?=w63:bool)
            n30 = Compound Arithmetic op=OR(w63, "Read Saved Config", w56) -> (w61:bool)
            n31 = case shown="True" w61 {
              tunnel: w57 -> [w87 w97]
              tunnel: [w87 w96] -> w60
              frame False {
              }
              frame True {
                w95 = TRUE ("Data Read")
                n32 = Unbundle By Name(w97) -> ("Team Files Folder"=w90:path, "AutoData"=w94:T32)
                n33 = call "RWA_File Config.vim"("Read(f) Write(t)"=FALSE, "Target Folder Folder"=w90, "Any Config"=w94) -> ("Error Out"=→"Error Out":errorcluster, "Found"=→"Found":bool, "Message Out"=→"Message Out":string, "Any Config Out"=w93:T32)  [unwired: 4 in, 1 out]
                n34 = Bundle By Name(cluster=w97, "AutoData"=w93, "Step Index"=0, "Data Read"=w95, "Update Display"=w95) -> (w96:T35)
              }
            }
          }
          frame "Autonomous Enabled" {
            # "Previously AUTO"
            n35 = Bundle By Name(cluster=w99, "Target Time (ms)"=u32 500) -> (w105:T35)
            n36 = Bundle By Name(cluster=w105, "CMD_ACT_SwerveDrive"=T21 {"Mode"=enum."Coast", "Direction"={"Traverse"={"Velocity"=0.0, "Angle"=0.0, "Rotations Count"=0.0}, "Rotate(Yaw) CCW 1 CW -1"=0.0}, "Orientation Robot(t) Field(f)"=FALSE, "Max Translation Speed (ft/sec)"=0.0, "Rotation Reduction 1-0"=0.0, "Rotation Center From Robot Center"={"X"=0.0, "Y"=0.0}, "Auto Angle"=0.0, "Auto Target (ft)"=0.0} ("CMD_ACT_Drive"), "CMD_ACT_Sholder"=T28 {"Mode"=enum."STOP", "Position (counts)"=0, "Velocity (0-1)"=0.0} ("CMD_ACT_Shooter"), "CMD_ACT_Grabber"=T20 {"Mode"=enum."STOP"} ("CMD_ACT_Intake"), "CMD_ACT_Extend"=T18 {"Mode"=enum."STOP", "Position (counts)"=0, "Velocity (0-1)"=0.0} ("CMD_ACT_Convayor"), "CMD_ACT_Wrist_Data"=T15 {"Mode"=enum."STOP", "Position (counts)"=0, "Velocity (0-1)"=0.0}) -> (w106:T35)
            n37 = Unbundle By Name(w106) -> ("CMD_ACT_Sholder"=w102:T28, "CMD_ACT_SwerveDrive"=w110:T21, "CMD_SEN_Pigeon_CMD"=w111:T14, "CMD_ACT_Grabber"=w112:T20, "CMD_ACT_Extend"=w113:T18, "CMD_ACT_Wrist_Data"=w101:T15)
            n38 = global write "Global_CMD_ACT_Data In.vi" "CMD_ACT_Sholder_Data"(w102) -> ()
            n39 = global write "Global_CMD_ACT_Data In.vi" "CMD_ACT_SwerveDrive_Data"(w110) -> ()
            n40 = global write "Global_CMD_SEN_Data In.vi" "CMD_SEN_Pigeon_Data"(w111) -> ()
            n41 = global write "Global_CMD_ACT_Data In.vi" "CMD_ACT_Grabber_Data"(w112) -> ()
            n42 = global write "Global_CMD_ACT_Data In.vi" "CMD_ACT_Extend_Data"(w113) -> ()
            n43 = global write "Global_CMD_ACT_Data In.vi" "CMD_ACT_Wrist Data"(w101) -> ()
          }
        }
      }
      frame "Autonomous Enabled" {
        # "AUTO"
        n44 = Unbundle By Name(w124) -> ("Current Time"=w134:timestamp)
        n45 = global read "Global_ACT_Data Out.vi" "ACT_SwerveDrive_Directions"() -> (w150:dbl[])
        n46 = global read "Global_ACT_Data Out.vi" "ACT_Sholder_SW Outputs"() -> (w155:T30)
        "Sholder_SW_Out" <- w155
        n47 = global read "Global_ACT_Data Out.vi" "ACT_SwerveDrive_At Position"() -> (w135:bool)
        "Drive At Position" <- w135
        n48 = global read "Global_ACT_Data Out.vi" "ACT_SwerveDrive_Balanced"() -> (w132:bool)
        "Balanced" <- w132
        n49 = global read "Global_ACT_Data Out.vi" "ACT_Grabber_SW Output"() -> (w152:T34)
        n50 = global read "Global_ACT_Data Out.vi" "ACT_Swerve_Position ft"() -> (w119:dbl)
        n51 = global read "Global_ACT_Data Out.vi" "ACT_Extend_SW Output"() -> (w147:T31)
        "Extend_SW_Out" <- w147
        n52 = global read "Global_CMD_CMD_Data In.vi" "CMD_CMD_2022-Auto_Data"() -> (w125:T17)
        "CMD_CMD_2022-Auto_Data" <- w125
        n53 = global read "Global_ACT_Data Out.vi" "ACT_Wrist_SW Output"() -> (w149:T13)
        "ACT_Wrist_SW Out" <- w149
        n54 = global read "Global_SEN_Data Out.vi" "Sen_Pigeon_Tilt Data"() -> (w123:T1)
        "Sen_Pigeon_Tilt Data" <- w123
        n55 = global read "Global_ACT_Data Out.vi" "ACT_SwerveDrive_At Angle"() -> (w136:bool)
        "Drive At Angle" <- w136
        n56 = call <vilib>:"WPI_DriverStationGetRemainingMatchTime.vi"() -> ("Match Time(s)"=w122:sgl)  [unwired: 10 in, 1 out]
        n57 = Bundle By Name(cluster=w124, "Swerve_Position ft"=w119, "Tilt Data"=w123, "Previous Time"=w134, "Current Time"=w170, "CMD Input"=w125, "Sholder_SW_Outputs"=w155, "SwerveDrive_Directions"=w150, "Grabber_SW_Out"=w152, "Wrist_SW_Out"=w149, "Drive At Position"=w135, "Extend_SW_Out"=w147, "At Angle Target"=w136, "Balanced"=w132, "Remaing Match Time"=w122) -> (w117:T35)
        n58 = Unbundle By Name(w117) -> ("Current Time"=w161:timestamp, "Previous Time"=w162:timestamp)
        n59 = Unbundle By Name(w117) -> ("State"=w165:T6, "Previous State"=w164:T6)
        n60 = Unbundle By Name(w117) -> ("Remaing Match Time"=w116:sgl)
        n61 = Subtract(x=w161, y=w162) -> (x-y=w159:dbl)
        n62 = Select(t=ENUM_CMD_State."Shutting Down" ("State"), s=w143, f=w165) -> (s? t:f=w163:T6)
        n63 = Bundle By Name(cluster=w117, "Cycle Time(S)"=w159) -> (w160:T35)
        n64 = Less?(x=w116, y=sgl 0.25) -> (x < y?=w114:bool)
        n65 = Build Array("Reset All", "Reset Sequence", w114) -> (w126:bool[])
        n66 = Or Array Elements(Boolean array=w126) -> (logical OR=w127:bool)
        n67 = case shown="\"Selecting Sequence\"" w163 {
          selector: w163 -> [_ _ w191 _ _ w251 w279 w307 w339 w363 _ w396 w429 w451 w471 _]
          tunnel: w160 -> [w179 w185 w187 w216 w237 w258 w286 w314 w346 w370 w388 w399 w427 w452 w472 w491]
          tunnel: [w180 w185 w186 w217 w240 w261 w289 w317 w349 w373 w389 w398 w431 w453 w473 w491] -> w168
          tunnel: [ENUM_CMD_State."Selecting Sequence" ("State") ENUM_CMD_State."Selecting Sequence" ("State") w189 w213 w239 w260 w288 w316 w348 w372 ENUM_CMD_State."Idling" ("State") w397 w430 w454 w474 ENUM_CMD_State."Shutting Down" ("State")] -> w167
          tunnel: [w182 w183 w193 w212 w238 _ _ _ _ _ _ _ _ _ _ w489] -> w158
          tunnel: w164 -> [_ _ w192 _ _ _ _ _ _ _ _ _ _ _ _ _]
          tunnel: "Set Manual" -> [_ _ _ _ _ _ _ _ _ _ _ _ _ _ _ _]
          frame "Starting" {
            w182 = T12[] [enum."Reset Time"] items=["No Action", "Reset Time", "Reset All", "Set System Cmds", "Reset Sequence", "Conveyor Off", "Config File Read", "Config File Wirte", "Config from FP", "Lock Wheels"] ("Actions")
            n68 = Bundle By Name(cluster=w179, "Target Time (ms)"=u32 50) -> (w180:T35)
          }
          frame "Configuring" {
            w183 = T12[] [enum."Config File Read"] items=["No Action", "Reset Time", "Reset All", "Set System Cmds", "Reset Sequence", "Conveyor Off", "Config File Read", "Config File Wirte", "Config from FP", "Lock Wheels"] ("Actions")
          }
          frame "Idling" {
            n69 = Unbundle By Name(w187) -> ("Robot Mode"=w190:T33, "Prev Robot Mode"=w188:T33)
            n70 = case shown="\"Autonomous Disabled\", Default" w190 {
              tunnel: [_ w201] -> w193
              tunnel: w192 -> [_ w200]
              tunnel: w191 -> [_ w199]
              tunnel: [ENUM_CMD_State."Stopping" ("State") w197] -> w189
              tunnel: w188 -> [_ w198]
              tunnel: w187 -> [w194 w196]
              tunnel: [w194 w196] -> w186
              frame "Autonomous Disabled", Default {
              }
              frame "Autonomous Enabled" {
                n71 = case shown="\"Autonomous Enabled\"" w198 {
                  tunnel: [w202 w208] -> w201
                  tunnel: w200 -> [_ w207]
                  tunnel: w199 -> [_ w206]
                  tunnel: [ENUM_CMD_State."Selecting Sequence" ("State") ENUM_CMD_State."Selecting Next Step" ("State")] -> w197
                  frame Default {
                    w202 = T12[] [enum."Reset All"] items=["No Action", "Reset Time", "Reset All", "Set System Cmds", "Reset Sequence", "Conveyor Off", "Config File Read", "Config File Wirte", "Config from FP", "Lock Wheels"] ("Actions")
                  }
                  frame "Autonomous Enabled" {
                    n72 = Not Equal?(x=w206, y=w207) -> (x != y?=w205:bool)
                    n73 = case shown="True" w205 {
                      tunnel: [_ w209] -> w208
                      frame False {
                      }
                      frame True {
                        w209 = T12[] [enum."Reset All"] items=["No Action", "Reset Time", "Reset All", "Set System Cmds", "Reset Sequence", "Conveyor Off", "Config File Read", "Config File Wirte", "Config from FP", "Lock Wheels"] ("Actions")
                      }
                    }
                  }
                }
              }
            }
          }
          frame "Selecting Sequence" {
            n74 = Unbundle By Name(w216) -> ("AutoData.Sequences"=w210:T4[], "CMD Input.Auto Select"=w218:T3)
            "CMD Input.Auto Select" <- w218
            n75 = case shown="\"Manual\"" w218 {
              selector: w218 -> [_ w220 _]
              tunnel: [_ w221 w229] -> w215
              tunnel: [ENUM_CMD_State."Stopping" ("State") ENUM_CMD_State."Selecting Next Step" ("State") ENUM_CMD_State."Selecting Next Step" ("State")] -> w213
              tunnel: [_ _ w231] -> w212
              tunnel: w210 -> [_ w222 _]
              frame "Unknown" {
              }
              frame Default {
                n76 = for {
                  tunnel: w222 -> [w228] mode=indexing
                  tunnel: w220 -> [w226]
                  tunnel: [w227] -> w221
                  stop <- w224 stop-if-true
                  n77 = Unbundle By Name(w228) -> ("Name"=w225:T3)
                  n78 = Equal?(x=w226, y=w225) -> (x = y?=w224:bool)
                  n79 = Unbundle By Name(w228) -> ("List"=w227:T5[])
                }
              }
              frame "Manual" {
                w231 = T12[] [enum."Reset All"] items=["No Action", "Reset Time", "Reset All", "Set System Cmds", "Reset Sequence", "Conveyor Off", "Config File Read", "Config File Wirte", "Config from FP", "Lock Wheels"] ("Actions")
                n80 = Build Array("Single Step") -> (w229:T5[])
              }
            }
            n81 = Bundle By Name(cluster=w216, "Sequence Array"=w215, "Step Index"=0, "Target Time (ms)"=u32 50) -> (w217:T35)
          }
          frame "Selecting Next Step" {
            n82 = Unbundle By Name(w237) -> ("Sequence Array"=w236:T5[], "Step Index"=w235:i32)
            n83 = Array Size(array=w236) -> (size(s)=w234:i32)
            n84 = Not Equal?(x=w234, y=w235) -> (x != y?=w233:bool)
            n85 = case shown="False" w233 {
              tunnel: [w242 w250] -> w240
              tunnel: w237 -> [w242 w248]
              tunnel: [ENUM_CMD_State."Stopping" ("State") w246] -> w239
              tunnel: [_ w245] -> w238
              tunnel: w236 -> [_ w244]
              tunnel: w235 -> [_ w243]
              frame False {
                # "End of sequence array"
              }
              frame True {
                w245 = T12[] [enum."Set System Cmds"] items=["No Action", "Reset Time", "Reset All", "Set System Cmds", "Reset Sequence", "Conveyor Off", "Config File Read", "Config File Wirte", "Config from FP", "Lock Wheels"] ("Actions")
                # "Not the end of sequece array"
                n86 = Index Array(array=w244, index=w243) -> (element=w249:T5)
                n87 = Unbundle By Name(w249) -> ("CMDs"=w247:T7, "State"=w246:T6)
                n88 = Bundle By Name(cluster=w248, "Step Data"=w247) -> (w250:T35)
              }
            }
          }
          frame "Driving to Position" {
            n89 = Unbundle By Name(w258) -> ("Current Time"=w264:timestamp, "Start Time"=w263:timestamp, "Sequence Array"=w267:T5[], "Step Index"=w266:i32)
            n90 = Unbundle By Name(w258) -> ("Drive At Position"=w253:bool)
            n91 = Subtract(x=w264, y=w263) -> (x-y=w262:dbl)
            n92 = Index Array(array=w267, index=w266) -> (element=w265:T5)
            n93 = Unbundle By Name(w265) -> ("Max Wait Time (S)"=w259:dbl)
            n94 = Greater Or Equal?(x=w262, y=w259) -> (x >= y?=w257:bool)
            n95 = feedback #1(FALSE) -> (w254:bool)
            n96 = feedback-in #1(w253) -> ()
            n97 = Greater?(x=w253, y=w254) -> (0:w252:bool)
            n98 = Or(x=w252, y=w257) -> (x .or. y?=w256:bool)
            n99 = case shown="True" w256 {
              tunnel: [w269 w272] -> w261
              tunnel: w258 -> [w269 w273]
              tunnel: [w268 ENUM_CMD_State."Selecting Next Step" ("State")] -> w260
              tunnel: w251 -> [w268 _]
              frame False {
                # "Not Complete"
              }
              frame True {
                # "Complete"
                n100 = Unbundle By Name(w273) -> ("Step Index"=w271:i32)
                n101 = Increment(x=w271) -> (x+1=w270:i32)
                n102 = Bundle By Name(cluster=w273, "Step Index"=w270) -> (w272:T35)
              }
            }
          }
          frame "Tilt UP or Position" {
            n103 = Unbundle By Name(w286) -> ("Current Time"=w292:timestamp, "Start Time"=w291:timestamp, "Sequence Array"=w295:T5[], "Step Index"=w294:i32)
            n104 = Unbundle By Name(w286) -> ("Tilt Data.BACK UP"=w276:bool, "Drive At Position"=w281:bool)
            n105 = Subtract(x=w292, y=w291) -> (x-y=w290:dbl)
            n106 = Index Array(array=w295, index=w294) -> (element=w293:T5)
            n107 = Unbundle By Name(w293) -> ("Max Wait Time (S)"=w287:dbl)
            n108 = call "Bool_Delay OnOFF.vi"("Delay Time(S)"=0.5, "Delay On(t) Off(f)"=TRUE, "Input"=w276) -> ("Output"=w275:bool)  [unwired: 7 in, 1 out]
            n109 = Greater Or Equal?(x=w290, y=w287) -> (x >= y?=w285:bool)
            n110 = feedback #2(FALSE) -> (w282:bool)
            n111 = feedback-in #2(w281) -> ()
            n112 = Greater?(x=w281, y=w282) -> (0:w280:bool)
            n113 = Compound Arithmetic op=OR(w275, w280, w285) -> (w284:bool)
            n114 = case shown="True" w284 {
              tunnel: [w297 w300] -> w289
              tunnel: w286 -> [w297 w301]
              tunnel: [w296 ENUM_CMD_State."Selecting Next Step" ("State")] -> w288
              tunnel: w279 -> [w296 _]
              frame False {
                # "Not Complete"
              }
              frame True {
                # "Complete"
                n115 = Unbundle By Name(w301) -> ("Step Index"=w299:i32)
                n116 = Increment(x=w299) -> (x+1=w298:i32)
                n117 = Bundle By Name(cluster=w301, "Step Index"=w298) -> (w300:T35)
              }
            }
          }
          frame "Tile DOWN or Position" {
            n118 = Unbundle By Name(w314) -> ("Current Time"=w320:timestamp, "Start Time"=w319:timestamp, "Sequence Array"=w323:T5[], "Step Index"=w322:i32)
            n119 = Unbundle By Name(w314) -> ("Tilt Data.BACK DOWN"=w304:bool, "Drive At Position"=w309:bool)
            n120 = Subtract(x=w320, y=w319) -> (x-y=w318:dbl)
            n121 = Index Array(array=w323, index=w322) -> (element=w321:T5)
            n122 = Unbundle By Name(w321) -> ("Max Wait Time (S)"=w315:dbl)
            n123 = Greater Or Equal?(x=w318, y=w315) -> (x >= y?=w313:bool)
            n124 = feedback #3(FALSE) -> (w310:bool)
            n125 = feedback-in #3(w309) -> ()
            n126 = call "Bool_Delay OnOFF.vi"("Delay Time(S)"=0.5, "Delay On(t) Off(f)"=TRUE, "Input"=w304) -> ("Output"=w303:bool)  [unwired: 7 in, 1 out]
            n127 = Greater?(x=w309, y=w310) -> (0:w308:bool)
            n128 = Compound Arithmetic op=OR(w303, w308, w313) -> (w312:bool)
            n129 = case shown="True" w312 {
              tunnel: [w325 w329] -> w317
              tunnel: w314 -> [w325 w326]
              tunnel: [w324 ENUM_CMD_State."Selecting Next Step" ("State")] -> w316
              tunnel: w307 -> [w324 _]
              frame False {
                # "Not Complete"
              }
              frame True {
                # "Complete"
                n130 = Unbundle By Name(w326) -> ("Step Index"=w328:i32)
                n131 = Increment(x=w328) -> (x+1=w327:i32)
                n132 = Bundle By Name(cluster=w326, "Step Index"=w327) -> (w329:T35)
              }
            }
          }
          frame "LEVEL or Position" {
            n133 = Unbundle By Name(w346) -> ("Current Time"=w352:timestamp, "Start Time"=w351:timestamp, "Sequence Array"=w355:T5[], "Step Index"=w354:i32)
            n134 = Unbundle By Name(w346) -> ("Tilt Data.BACK UP"=w338:bool, "Tilt Data.BACK DOWN"=w337:bool, "Drive At Position"=w341:bool)
            n135 = Subtract(x=w352, y=w351) -> (x-y=w350:dbl)
            n136 = Index Array(array=w355, index=w354) -> (element=w353:T5)
            n137 = Not(x=w338) -> (.not. x?=w336:bool)
            n138 = Not(x=w337) -> (.not. x?=w335:bool)
            n139 = Unbundle By Name(w353) -> ("Max Wait Time (S)"=w347:dbl)
            n140 = Greater Or Equal?(x=w350, y=w347) -> (x >= y?=w345:bool)
            n141 = And(x=w336, y=w335) -> (x .and. y?=w332:bool)
            n142 = feedback #4(FALSE) -> (w342:bool)
            n143 = feedback-in #4(w341) -> ()
            n144 = Greater?(x=w341, y=w342) -> (0:w340:bool)
            n145 = call "Bool_Delay OnOFF.vi"("Delay Time(S)"=0.5, "Delay On(t) Off(f)"=TRUE, "Input"=w332) -> ("Output"=w331:bool)  [unwired: 7 in, 1 out]
            n146 = Compound Arithmetic op=OR(w331, w340, w345) -> (w344:bool)
            n147 = case shown="True" w344 {
              tunnel: [w357 w360] -> w349
              tunnel: w346 -> [w357 w361]
              tunnel: [w356 ENUM_CMD_State."Selecting Next Step" ("State")] -> w348
              tunnel: w339 -> [w356 _]
              frame False {
                # "Not Complete"
              }
              frame True {
                # "Complete"
                n148 = Unbundle By Name(w361) -> ("Step Index"=w359:i32)
                n149 = Increment(x=w359) -> (x+1=w358:i32)
                n150 = Bundle By Name(cluster=w361, "Step Index"=w358) -> (w360:T35)
              }
            }
          }
          frame "Balancing Level" {
            n151 = Unbundle By Name(w370) -> ("Current Time"=w376:timestamp, "Start Time"=w375:timestamp, "Sequence Array"=w379:T5[], "Step Index"=w378:i32)
            n152 = Unbundle By Name(w370) -> ("Balanced"=w365:bool)
            n153 = Subtract(x=w376, y=w375) -> (x-y=w374:dbl)
            n154 = Index Array(array=w379, index=w378) -> (element=w377:T5)
            n155 = Unbundle By Name(w377) -> ("Max Wait Time (S)"=w371:dbl)
            n156 = Greater Or Equal?(x=w374, y=w371) -> (x >= y?=w369:bool)
            n157 = feedback #5(FALSE) -> (w366:bool)
            n158 = feedback-in #5(w365) -> ()
            n159 = Greater?(x=w365, y=w366) -> (0:w364:bool)
            n160 = Or(x=w364, y=w369) -> (x .or. y?=w368:bool)
            n161 = case shown="True" w368 {
              tunnel: [w381 w384] -> w373
              tunnel: w370 -> [w381 w385]
              tunnel: [w380 ENUM_CMD_State."Selecting Next Step" ("State")] -> w372
              tunnel: w363 -> [w380 _]
              frame False {
                # "Not Complete"
              }
              frame True {
                # "Complete"
                n162 = Unbundle By Name(w385) -> ("Step Index"=w383:i32)
                n163 = Increment(x=w383) -> (x+1=w382:i32)
                n164 = Bundle By Name(cluster=w385, "Step Index"=w382) -> (w384:T35)
              }
            }
          }
          frame "Stopping" {
            n165 = Bundle By Name(cluster=w388, "CMD_ACT_SwerveDrive"=T21 {"Mode"=enum."Coast", "Direction"={"Traverse"={"Velocity"=0.0, "Angle"=0.0, "Rotations Count"=0.0}, "Rotate(Yaw) CCW 1 CW -1"=0.0}, "Orientation Robot(t) Field(f)"=FALSE, "Max Translation Speed (ft/sec)"=0.0, "Rotation Reduction 1-0"=0.0, "Rotation Center From Robot Center"={"X"=0.0, "Y"=0.0}, "Auto Angle"=0.0, "Auto Target (ft)"=0.0} ("CMD_ACT_Drive"), "CMD_ACT_Sholder"=T28 {"Mode"=enum."STOP", "Position (counts)"=0, "Velocity (0-1)"=0.0} ("CMD_ACT_Shooter"), "CMD_ACT_Grabber"=T20 {"Mode"=enum."STOP"} ("CMD_ACT_Intake"), "CMD_ACT_Extend"=T18 {"Mode"=enum."STOP", "Position (counts)"=0, "Velocity (0-1)"=0.0} ("CMD_ACT_Convayor"), "CMD_ACT_Wrist_Data"=T15 {"Mode"=enum."STOP", "Position (counts)"=0, "Velocity (0-1)"=0.0}) -> (w389:T35)
          }
          frame "Grabbing" {
            n166 = Unbundle By Name(w399) -> ("Current Time"=w403:timestamp, "Start Time"=w402:timestamp, "Sequence Array"=w406:T5[], "Step Index"=w405:i32)
            n167 = Index Array(array=w406, index=w405) -> (element=w404:T5)
            n168 = Unbundle By Name(w404) -> ("Max Wait Time (S)"=w400:dbl)
            n169 = Subtract(x=w403, y=w402) -> (x-y=w401:dbl)
            n170 = Greater Or Equal?(x=w401, y=w400) -> (x >= y?=w395:bool)
            n171 = case shown="False" w395 {
              tunnel: [w408 w411] -> w398
              tunnel: w399 -> [w408 w412]
              tunnel: [w407 ENUM_CMD_State."Selecting Next Step" ("State")] -> w397
              tunnel: w396 -> [w407 _]
              frame False {
                # "Not Complete"
              }
              frame True {
                # "Complete"
                n172 = Unbundle By Name(w412) -> ("Step Index"=w410:i32)
                n173 = Increment(x=w410) -> (x+1=w409:i32)
                n174 = Bundle By Name(cluster=w412, "Step Index"=w409) -> (w411:T35)
              }
            }
          }
          frame "Moving Arm" {
            w420 = TRUE ("Initial State")
            # "Rising edge\nand All 3 \ncomplete"
            # "Any axis completes"
            n175 = Unbundle By Name(w427) -> ("Sholder_SW_Outputs.At Positon"=w426:bool, "Extend_SW_Out.exAt Positon"=w425:bool, "Wrist_SW_Out.Wr At Positon"=w424:bool)
            n176 = Unbundle By Name(w427) -> ("Current Time"=w435:timestamp, "Start Time"=w434:timestamp, "Sequence Array"=w438:T5[], "Step Index"=w437:i32)
            n177 = Index Array(array=w438, index=w437) -> (element=w436:T5)
            n178 = Unbundle By Name(w436) -> ("Max Wait Time (S)"=w432:dbl)
            n179 = call "Bool_Edge Detect.vi"("Initial State"=w420, "Input/Set"=w426) -> ("Rise"=w421:bool, "Output"=w418:bool)  [unwired: 6 in, 2 out]
            n180 = call "Bool_Edge Detect.vi"("Initial State"=w420, "Input/Set"=w425) -> ("Rise"=w422:bool, "Output"=w417:bool)  [unwired: 6 in, 2 out]
            n181 = call "Bool_Edge Detect.vi"("Initial State"=w420, "Input/Set"=w424) -> ("Rise"=w423:bool, "Output"=w416:bool)  [unwired: 6 in, 2 out]
            n182 = Subtract(x=w435, y=w434) -> (x-y=w433:dbl)
            n183 = Compound Arithmetic op=OR(w421, w422, w423) -> (w419:bool)
            n184 = Compound Arithmetic op=AND(w419, w418, w417, w416) -> (w414:bool)
            n185 = Greater Or Equal?(x=w433, y=w432) -> (x >= y?=w428:bool)
            n186 = Or(x=w414, y=w428) -> (x .or. y?=w415:bool)
            n187 = case shown="True" w415 {
              tunnel: [w440 w443] -> w431
              tunnel: w427 -> [w440 w444]
              tunnel: [w439 ENUM_CMD_State."Selecting Next Step" ("State")] -> w430
              tunnel: w429 -> [w439 _]
              frame False {
                # "Not Complete"
              }
              frame True {
                # "Complete"
                n188 = Unbundle By Name(w444) -> ("Step Index"=w442:i32)
                n189 = Increment(x=w442) -> (x+1=w441:i32)
                n190 = Bundle By Name(cluster=w444, "Step Index"=w441) -> (w443:T35)
              }
            }
          }
          frame "Rotation Target" {
            n191 = Unbundle By Name(w452) -> ("Current Time"=w458:timestamp, "Start Time"=w459:timestamp, "Sequence Array"=w455:T5[], "Step Index"=w456:i32)
            n192 = Unbundle By Name(w452) -> ("At Angle Target"=w447:bool)
            n193 = Index Array(array=w455, index=w456) -> (element=w457:T5)
            n194 = Unbundle By Name(w457) -> ("Max Wait Time (S)"=w461:dbl)
            n195 = feedback-in #6(w447) -> ()
            n196 = feedback #6(FALSE) -> (w448:bool)
            n197 = Subtract(x=w458, y=w459) -> (x-y=w460:dbl)
            n198 = Greater?(x=w447, y=w448) -> (0:w446:bool)
            n199 = Greater Or Equal?(x=w460, y=w461) -> (x >= y?=w462:bool)
            n200 = Or(x=w446, y=w462) -> (x .or. y?=w450:bool)
            n201 = case shown="False" w450 {
              tunnel: [w463 ENUM_CMD_State."Selecting Next Step" ("State")] -> w454
              tunnel: [w464 w465] -> w453
              tunnel: w452 -> [w464 w466]
              tunnel: w451 -> [w463 _]
              frame False {
              }
              frame True {
                n202 = Unbundle By Name(w466) -> ("Step Index"=w469:i32)
                n203 = Increment(x=w469) -> (x+1=w468:i32)
                n204 = Bundle By Name(cluster=w466, "Step Index"=w468) -> (w465:T35)
              }
            }
          }
          frame "Waiting" {
            n205 = Unbundle By Name(w472) -> ("Current Time"=w478:timestamp, "Start Time"=w479:timestamp, "Sequence Array"=w475:T5[], "Step Index"=w476:i32)
            n206 = Index Array(array=w475, index=w476) -> (element=w477:T5)
            n207 = Unbundle By Name(w477) -> ("Max Wait Time (S)"=w481:dbl)
            n208 = Subtract(x=w478, y=w479) -> (x-y=w480:dbl)
            n209 = Greater Or Equal?(x=w480, y=w481) -> (x >= y?=w470:bool)
            n210 = case shown="True" w470 {
              tunnel: [w482 ENUM_CMD_State."Selecting Next Step" ("State")] -> w474
              tunnel: [w483 w484] -> w473
              tunnel: w472 -> [w483 w485]
              tunnel: w471 -> [w482 _]
              frame False {
              }
              frame True {
                n211 = Unbundle By Name(w485) -> ("Step Index"=w488:i32)
                n212 = Increment(x=w488) -> (x+1=w487:i32)
                n213 = Bundle By Name(cluster=w485, "Step Index"=w487) -> (w484:T35)
              }
            }
          }
          frame "Shutting Down" {
            w489 = T12[] [enum."Reset All"] items=["No Action", "Reset Time", "Reset All", "Set System Cmds", "Reset Sequence", "Conveyor Off", "Config File Read", "Config File Wirte", "Config from FP", "Lock Wheels"] ("Actions")
          }
        }
        "State" <- w167
        n214 = case shown="True" w127 {
          tunnel: [_ w174] -> w145
          tunnel: w126 -> [_ w173]
          frame False {
          }
          frame True {
            n215 = call "Search Unsorted 1D Array.vim"("element"=TRUE, "unsorted 1D array"=w173) -> ("index of element"=w171:i32)  [unwired: 9 in]
            n216 = case shown="2.." w171 {
              tunnel: [w175 w176 w177] -> w174
              frame ..0 {
                w175 = T12[] [enum."Reset All"] items=["No Action", "Reset Time", "Reset All", "Set System Cmds", "Reset Sequence", "Conveyor Off", "Config File Read", "Config File Wirte", "Config from FP", "Lock Wheels"] ("Actions")
                # "Reset All"
              }
              frame 1 {
                w176 = T12[] [enum."Reset Sequence"] items=["No Action", "Reset Time", "Reset All", "Set System Cmds", "Reset Sequence", "Conveyor Off", "Config File Read", "Config File Wirte", "Config from FP", "Lock Wheels"] ("Actions")
                # "Reset Sequence"
              }
              frame 2.. {
                w177 = T12[] [enum."Lock Wheels"] items=["No Action", "Reset Time", "Reset All", "Set System Cmds", "Reset Sequence", "Conveyor Off", "Config File Read", "Config File Wirte", "Config from FP", "Lock Wheels"] ("Actions")
                # "Reset Sequence"
              }
            }
          }
        }
        n217 = Bundle By Name(cluster=w168, "Previous State"=w163, "State"=w167) -> (w169:T35)
        n218 = Build Array (concatenate)(w158, w145) -> (w146:T12[])
        n219 = for {
          tunnel: w146 -> [w494] mode=indexing
          shift-right: [w493] -> w121
          shift-left: w169 -> [w492]
          n220 = case shown="\"Lock Wheels\"" w494 {
            tunnel: w492 -> [w495 w498 w507 w511 w512 w518 w521 w526 w532 w536]
            tunnel: [w495 w497 w508 w510 w512 w519 w522 w527 w533 w536] -> w493
            frame "No Action" {
            }
            frame "Reset Time" {
              # "Reset timer by taking the current time\nand making it the start time\n\nLater when the current time is \nsubtracted from the start time\nyou will get the elapsed time in \nseconds"
              n221 = Unbundle By Name(w498) -> ("Current Time"=w496:timestamp)
              n222 = Bundle By Name(cluster=w498, "Start Time"=w496) -> (w497:T35)
            }
            frame "Set System Cmds" {
              n223 = Unbundle By Name(w507) -> ("Current Time"=w502:timestamp, "Step Data"=w506:T7, "Remaing Match Time"=w499:sgl)
              n224 = call "Sequence Data to Sytem CMDs.vi"("Remaining Match Time"=w499, "Sequence Data"=w506) -> ("CMD_ACT_Wrist_Data Out"=w500:T15, "CMD_ACT_Grabber_Data Out"=w505:T20, "CMD_ACT_Shooter_Data Out"=w501:T28, "CMD_ACT_Drive_Data Out"=w503:T21, "CMD_ACT_Extend Out"=w504:T18)  [unwired: 4 in, 1 out]
              n225 = Bundle By Name(cluster=w507, "Start Time"=w502, "CMD_ACT_SwerveDrive"=w503, "CMD_ACT_Sholder"=w501, "CMD_ACT_Grabber"=w505, "CMD_ACT_Wrist_Data"=w500, "CMD_ACT_Extend"=w504) -> (w508:T35)
            }
            frame "Lock Wheels" {
              n226 = Bundle By Name(cluster=w511, "CMD_ACT_SwerveDrive.Mode"=ENUM_Swerve_CMD_Mode_Select."Lock Wheels") -> (w510:T35)
            }
            frame "Conveyor Off" {
            }
            frame "Reset All" {
              n227 = Bundle By Name(cluster=w518, "CMD_ACT_SwerveDrive"=T21 {"Mode"=enum."Coast", "Direction"={"Traverse"={"Velocity"=0.0, "Angle"=0.0, "Rotations Count"=0.0}, "Rotate(Yaw) CCW 1 CW -1"=0.0}, "Orientation Robot(t) Field(f)"=FALSE, "Max Translation Speed (ft/sec)"=0.0, "Rotation Reduction 1-0"=0.0, "Rotation Center From Robot Center"={"X"=0.0, "Y"=0.0}, "Auto Angle"=0.0, "Auto Target (ft)"=0.0} ("CMD_ACT_Drive"), "CMD_ACT_Sholder"=T28 {"Mode"=enum."STOP", "Position (counts)"=0, "Velocity (0-1)"=0.0} ("CMD_ACT_Shooter"), "CMD_ACT_Grabber"=T20 {"Mode"=enum."STOP"} ("CMD_ACT_Intake"), "CMD_ACT_Extend"=T18 {"Mode"=enum."STOP", "Position (counts)"=0, "Velocity (0-1)"=0.0} ("CMD_ACT_Convayor"), "CMD_ACT_Wrist_Data"=T15 {"Mode"=enum."STOP", "Position (counts)"=0, "Velocity (0-1)"=0.0}) -> (w519:T35)
            }
            frame "Reset Sequence" {
              n228 = Bundle By Name(cluster=w521, "State"=ENUM_CMD_State."Selecting Sequence") -> (w522:T35)
            }
            frame "Config File Read" {
              n229 = Unbundle By Name(w526) -> ("Team Files Folder"=w528:path, "AutoData"=w529:T32)
              n230 = call "RWA_File Config.vim"("Read(f) Write(t)"=FALSE, "Target Folder Folder"=w528, "Any Config"=w529) -> ("Any Config Out"=w525:T32)  [unwired: 4 in, 4 out]
              n231 = Bundle By Name(cluster=w526, "AutoData"=w525, "Step Index"=0) -> (w527:T35)
            }
            frame "Config File Wirte" {
              n232 = Unbundle By Name(w532) -> ("Team Files Folder"=w534:path, "AutoData"=w535:T32)
              n233 = call "RWA_File Config.vim"("Read(f) Write(t)"=TRUE, "Target Folder Folder"=w534, "Any Config"=w535) -> ("Any Config Out"=w531:T32)  [unwired: 4 in, 4 out]
              n234 = Bundle By Name(cluster=w532, "AutoData"=w531) -> (w533:T35)
            }
            frame "Config from FP" {
            }
          }
          "Action" <- w494
        }
        n235 = Unbundle By Name(w121) -> ("Remaing Match Time"=→"Remaing Match Time":sgl)
        n236 = Unbundle By Name(w121) -> ("Sequence Array"=w142:T5[], "Step Index"=w141:i32)
        "Step Index 2" <- w141
        n237 = Unbundle By Name(w121) -> ("CMD_ACT_Wrist_Data"=w133:T15, "CMD_ACT_Sholder"=w137:T28, "CMD_ACT_SwerveDrive"=w154:T21, "CMD_SEN_Pigeon_CMD"=w153:T14, "CMD_ACT_Grabber"=w151:T20, "CMD_ACT_Extend"=w148:T18, "Step Index"=→"Step Index":i32, "Swerve_Position ft"=→"Swerve_Position ft":dbl)
        "CMD_ACT_Shooter" <- w137
        "CMD_ACT_Drive" <- w154
        "CMD_ACT_Grabber" <- w151
        "CMD_ACT_Extend" <- w148
        "CMD_ACT_Wrist" <- w133
        "CMD_SEN_Pigeon_CMD" <- w153
        n238 = Unbundle By Name(w121) -> ("Cycle Time(S)"=w156:dbl)
        "Cycle Time (S)" <- w156
        n239 = Unbundle By Name(w121) -> ("CMD Input"=→"Input Data":T17)
        n240 = Index Array(array=w142, index=w141) -> (element=w139:T5)
        n241 = call "Is Value Changed.vim"("value"=w139) -> ("changed or first call?"=w140:bool)
        n242 = global write "Global_CMD_Data Out.vi" "CMD_Template_CycleTime(S)"(w156) -> ()
        n243 = case shown="True" w140 {
          tunnel: w139 -> [_ w539]
          frame False {
          }
          frame True {
            n244 = local write "Single Step"(w539) -> ()
            n245 = global write "Global_CMD_Data Out.vi" "Single Step"(w539) -> ()
            n246 = Unbundle By Name(w539) -> ("Color Box"=w537:u32)
            n247 = call "NTV_AutoStepcolor.vi"("Read(f) Write(t)"=TRUE, "Color"=w537) -> ()  [unwired: 9 in, 1 out]
          }
        }
        n248 = global write "Global_CMD_ACT_Data In.vi" "CMD_ACT_Sholder_Data"(w137) -> ()
        n249 = global write "Global_CMD_ACT_Data In.vi" "CMD_ACT_SwerveDrive_Data"(w154) -> ()
        n250 = global write "Global_CMD_SEN_Data In.vi" "CMD_SEN_Pigeon_Data"(w153) -> ()
        n251 = global write "Global_CMD_ACT_Data In.vi" "CMD_ACT_Grabber_Data"(w151) -> ()
        n252 = global write "Global_CMD_ACT_Data In.vi" "CMD_ACT_Extend_Data"(w148) -> ()
        n253 = global write "Global_CMD_ACT_Data In.vi" "CMD_ACT_Wrist Data"(w133) -> ()
        n254 = Bundle By Name(cluster=w121, "Update Display"=FALSE) -> (w131:T35)
      }
    }
    n255 = Unbundle By Name(w42) -> ("AutoData.Sequences"=w44:T4[], "Update Display"=w43:bool)
    n256 = Bundle By Name(cluster=w42, "Update Display"=FALSE) -> (w41:T35)
    n257 = case shown="True" w43 {
      tunnel: w44 -> [_ w52]
      frame False {
      }
      frame True {
        n258 = local write "Sequences"(w52) -> ()
      }
    }
  }
  n259 = flat-sequence {
    frame #0 {
      (unwired) ENUM_CMD_State."Starting" ("State")
      (unwired) ENUM_CMD_Action."No Action" ("Action")
      # "State LIST"
      # "Action LIST"
    }
  }
